vi "UMLEditor reversedEngineering.vi"(1 "AddProjectClasses":bool, 2 "ClassToAnalyse/XMI File To Read":path, 3 "XMI Import":bool, 5 "error in (no error)":errorcluster) -> (16 "cancel":bool, 17 "newCLassDiagram":refnum<class "Graph.lvclass">, 19 "error out":errorcluster)   [LabVIEW 2020]
doc: "Gets current diagram values"
uses:
  <resource>/Framework/Providers/Open_GDS/UML/UMLEditor/UMLEditor RevEngLocalvarType.ctl
  <resource>/Framework/Providers/Open_GDS/UML/Graph_class/Graph.lvclass
  <resource>/Framework/Providers/Open_GDS/UML/Graphics_class/Graphics.lvclass
  <resource>/Framework/Providers/Open_GDS/UML/Grid_class/Grid.lvclass
  <resource>/Framework/Providers/Open_GDS/UML/ClassNode_class/ClassNode.lvclass
  C:/Program Files (x86)/National Instruments/LabVIEW 2020/resource/Framework/Providers/Open_GDS/UML/RectangularNode_class/RectangularNode.lvclass
  C:/Program Files (x86)/National Instruments/LabVIEW 2020/resource/Framework/Providers/Open_GDS/UML/AbstractNode_class/AbstractNode.lvclass
  <resource>/Framework/Providers/Open_GDS/UML/AbstractEdge_class/AbstractEdge.lvclass
  <resource>/Framework/Providers/Open_GDS/UML/AbstractNode_class/AbstractNode.lvclass
  <resource>/Framework/Providers/Open_GDS/UML/ReversedEngineering/ReversedEngineering ClassInfoType.ctl
  <resource>/Framework/Providers/Open_GDS/UML/UMLEditor/UMLEditor_VisibilityType.ctl
  <resource>/Framework/Providers/Open_GDS/UML/ReversedEngineering/ReversedEngineering AttributeInfoType.ctl
  <resource>/Framework/Providers/Open_GDS/ClassProviders/Common/CommonVIs/CommonVIs_AttributeDataType.ctl
  <resource>/Framework/Providers/Open_GDS/UML/ReversedEngineering/ReversedEngineering_ClassDependencyDetailsType.ctl
  <resource>/Framework/Providers/Open_GDS/ClassProviders/Common/ScriptingFunctions/SubVIs/Scripting_ViDependencyType.ctl
  <resource>/Framework/Providers/Open_GDS/UML/General/Rectangle/Rectangle Rectangle2D.ctl
  <resource>/Framework/Providers/Open_GDS/UML/ReversedEngineering/ReversedEngineering TypeDefType.ctl
  <resource>/Framework/Providers/Open_GDS/UML/ReversedEngineering/ReversedEngineering RecursiveSearchElements.ctl
  <resource>/Framework/Providers/Open_GDS/UML/UMLEditor/UMLEditor_SyncOptions.ctl
  <resource>/Framework/Providers/Open_GDS/UML/UMLEditor/UMLEditor GOOPWizardClassSpecification.ctl
  <resource>/Framework/Providers/Open_GDS/UML/Graphics_class/FontType.ctl
  <resource>/Framework/Providers/Open_GDS/UML/UMLEditor/UMLEditor BusyDialogAction.ctl
  <resource>/Framework/Providers/Open_GDS/UML/ContextHelp/ContextHelp_HelpTexts.ctl
  <resource>/Framework/Providers/Open_GDS/UML/UMLEditor/UMLEditor_StoredPathes.ctl
  <resource>/Framework/Providers/Open_GDS/ClassProviders/Common/File/File_StoredPathesActions.ctl
  <resource>/Framework/Providers/Open_GDS/UML/ClassNode_class/ExternalSetTypes.ctl
  <resource>/Framework/Providers/Open_GDS/UML/ClassRelationshipEdge_class/ExternaSetParamType.ctl
  <resource>/Framework/Providers/Open_GDS/UML/ArrowHead_class/ArrowHeadType.ctl
  <resource>/Framework/Providers/Open_GDS/UML/BentStyle_class/BentStyleType.ctl
  <resource>/Framework/Providers/Open_GDS/UML/Graphics_class/LvFontType.ctl
  <resource>/Framework/Providers/Open_GDS/UML/SegmentedLineEdge_class/SegmentedLineEdge.lvclass
  <resource>/Framework/Providers/Open_GDS/UML/InterfaceNode_class/InterfaceNode.lvclass
  C:/Program Files (x86)/National Instruments/LabVIEW 2020/resource/Framework/Providers/Open_GDS/UML/ClassNode_class/ClassNode.lvclass
  <resource>/Framework/Providers/Open_GDS/UML/ClassRelationshipEdge_class/ClassRelationshipEdge.lvclass
  C:/Program Files (x86)/National Instruments/LabVIEW 2020/resource/Framework/Providers/Open_GDS/UML/AbstractEdge_class/AbstractEdge.lvclass
  <resource>/Framework/Providers/Open_GDS/UML/ClassDiagramGraph_class/ClassDiagramGraph.lvclass
  C:/Program Files (x86)/National Instruments/LabVIEW 2020/resource/Framework/Providers/Open_GDS/UML/Graph_class/Graph.lvclass
  <resource>/Framework/Providers/Open_GDS/UML/ArrowHead_class/ArrowHead.lvclass
  <resource>/Framework/Providers/Open_GDS/UML/BentStyle_class/BentStyle.lvclass
  <resource>/Framework/Providers/Open_GDS/UML/RectangularNode_class/RectangularNode.lvclass
  <resource>/Framework/Providers/Open_GDS/UML/UmlEditor_class/UmlEditor.lvclass
panel:
  in  "SyncOption":T1
  in  "AddDirsRec":bool
  in  "ReverseCurrectProject":bool
  out "SearchElements":T2[](array[typedef])
  in  "Remove":bool
  in  "ClearList":bool
  in  "AddDirs":bool
  in  "AddClasses":bool
  in  "AddTopVIs":bool
  in  "Pathes":i32[](listbox) caption="Top VIs, Classes(llbs/dirs) and Directories that should be analysed"
  out "ApplicationNodes":i32[](array[numeric])
  in  "CreateApplication":bool caption="Create Main Application Node"
  in  "Help":bool
  in  "OnlyInheritance":bool caption="Only Create Inheritance classes"
  in  "CreateTypes":bool caption="Create TypeDefs"
  in  "HideSubAss":bool=TRUE caption="Hide SubClass assosiates to classes that BaseClass already associates to"
  in  "screenRef":refnum<vi>
  out "files":path[](array[path])
  in  "cancel":bool
  in  "ok":bool
  in  "local":T3 {"block"."bounds"."height" format="%.2f"; "block"."bounds"."width" format="%.2f"; "block"."bounds"."y" format="%.2f"; "block"."bounds"."x" format="%.2f"; "bounds"."height" format="%.2f"; "bounds"."width" format="%.2f"; "bounds"."y" format="%.2f"; "bounds"."x" format="%.2f"}
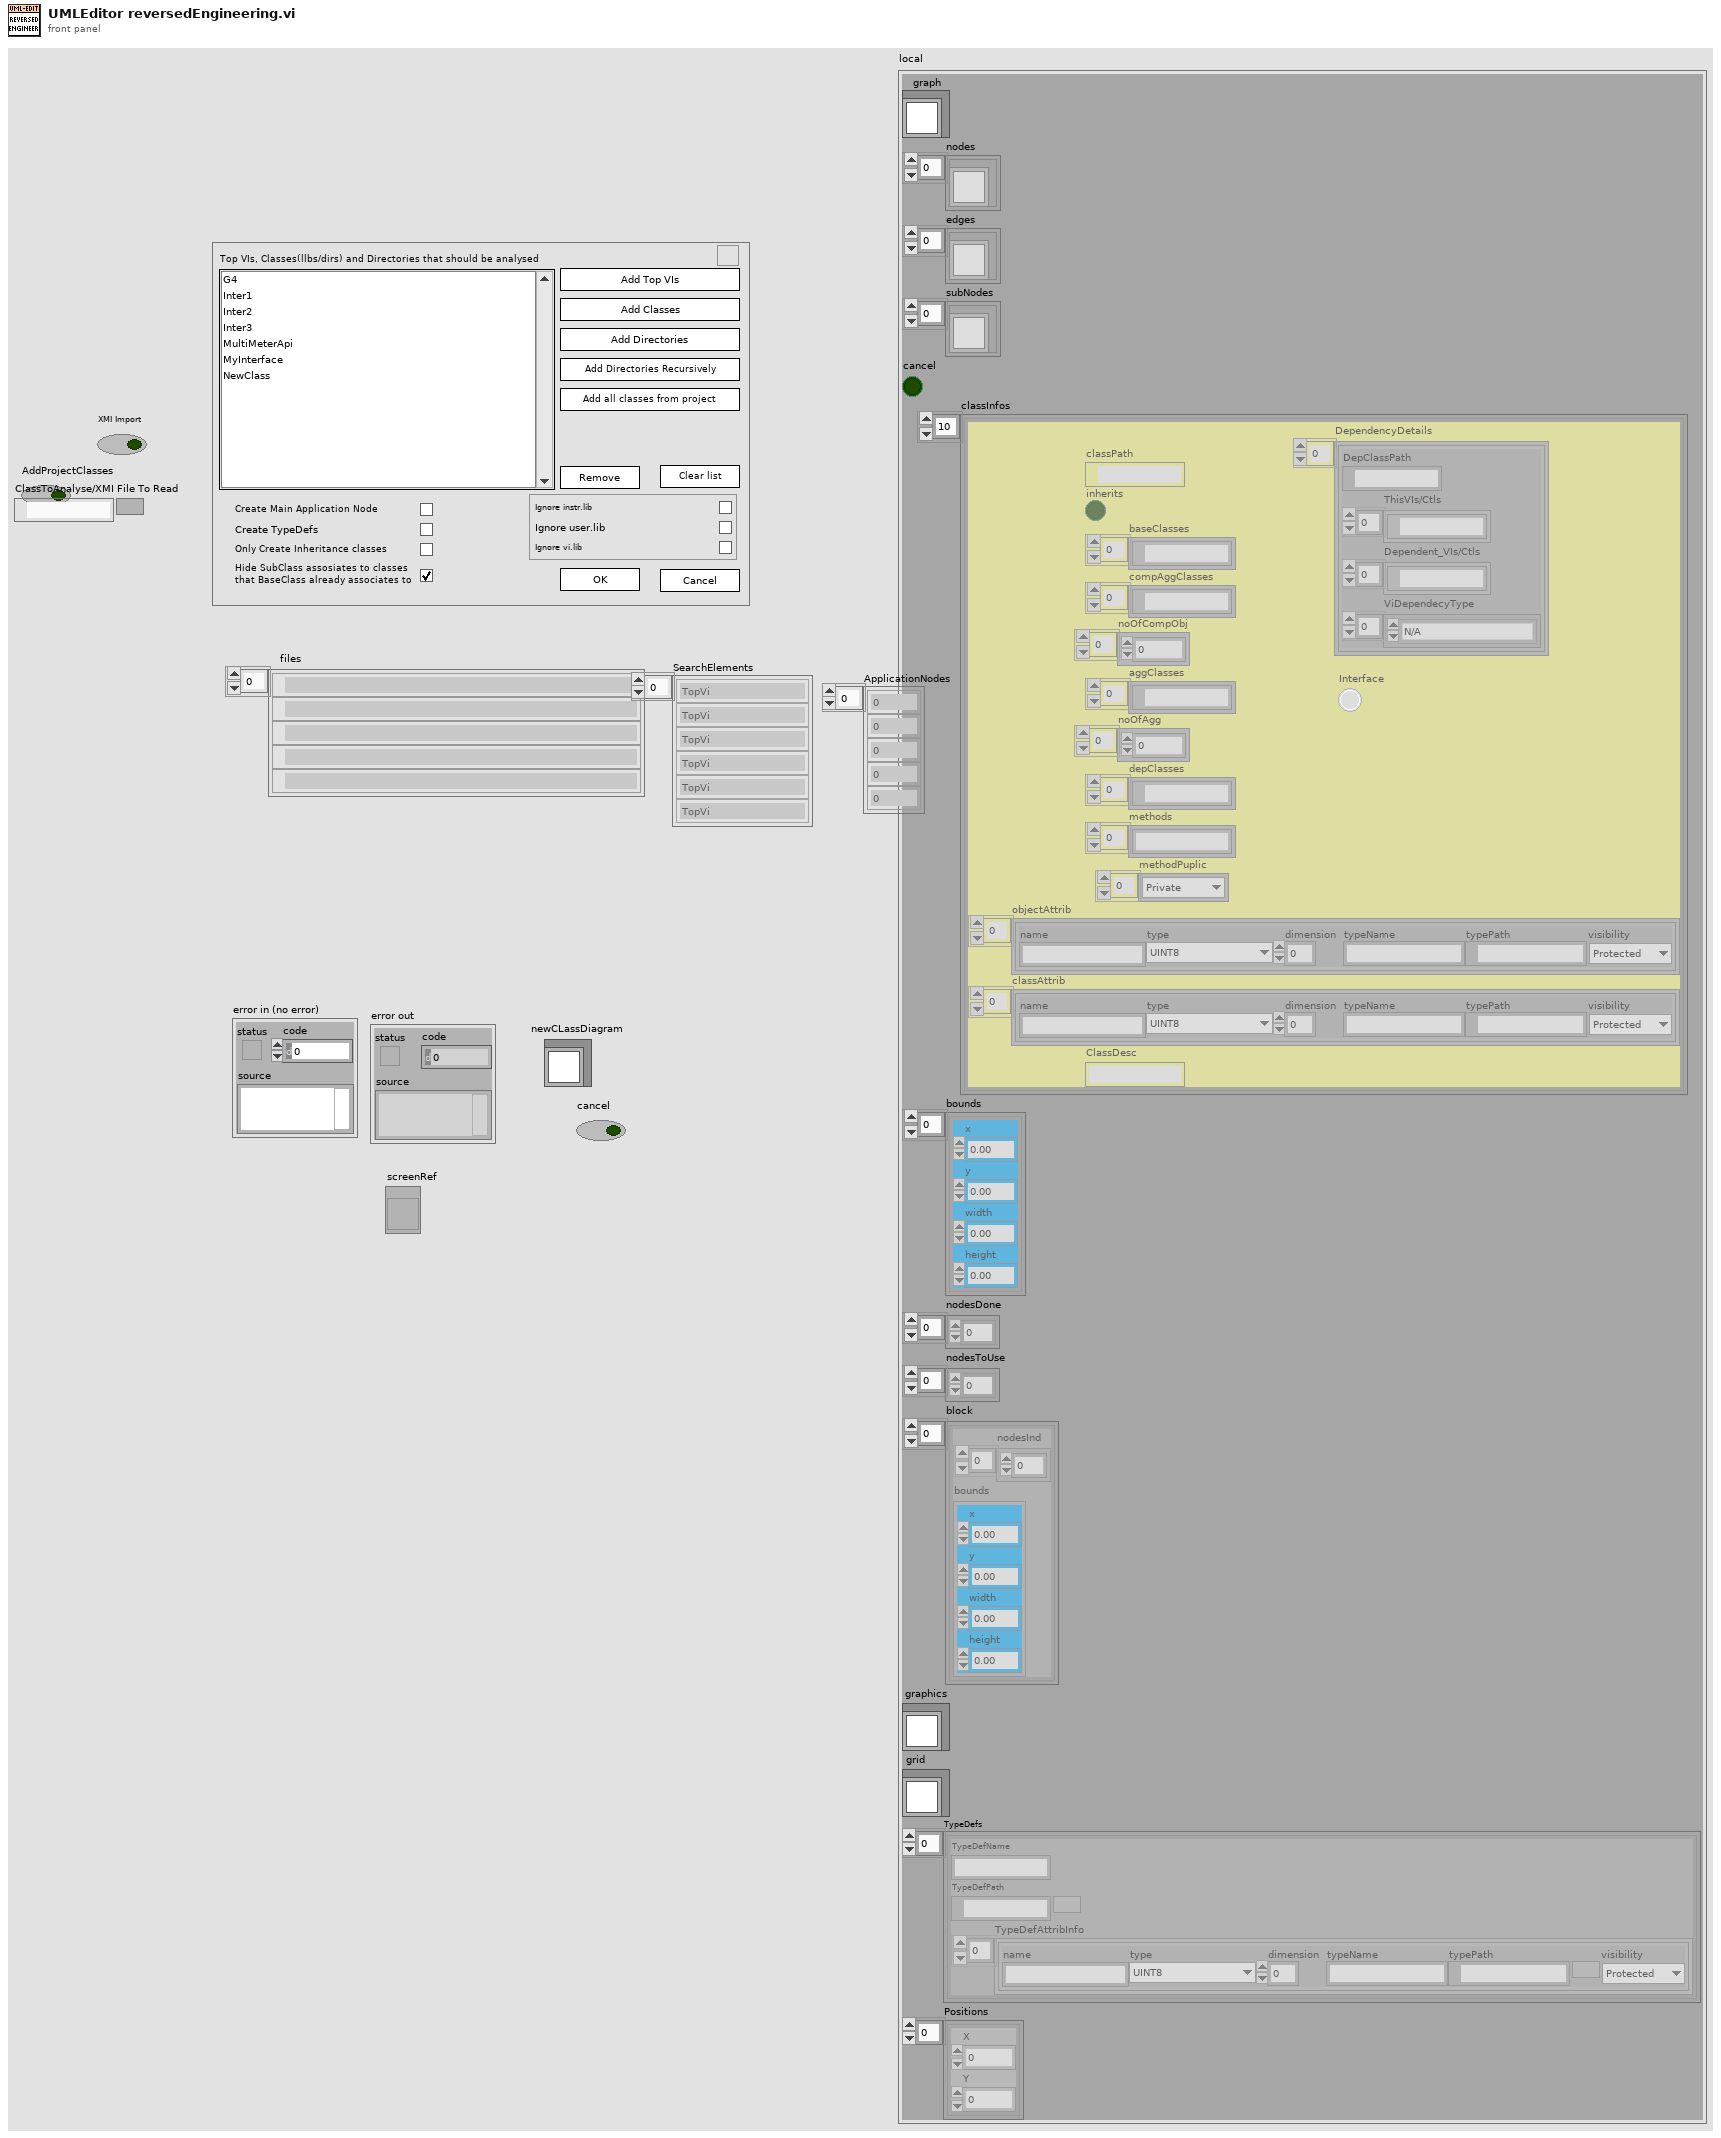
[diagram p1: front panel]
types:
  T1 = typedef "UMLEditor_SyncOptions.ctl" = cluster{"IgnoreInstrLib":bool, "IgnoreUserLib":bool, "IgnoreViLib":bool}
  T2 = typedef "ReversedEngineering RecursiveSearchElements.ctl" = enum16{"TopVi", "Class", "Dir", "Dir(rec.)"}
  T3 = typedef "UMLEditor RevEngLocalvarType.ctl" = cluster{"graph":refnum<class "Graph.lvclass">, "nodes":refnum<class "ClassNode.lvclass">[], "edges":refnum<class "AbstractEdge.lvclass">[], "subNodes":refnum<class "AbstractNode.lvclass">[], "cancel":bool, "classInfos":T4[], "bounds":T10[], "nodesDone":i32[], "nodesToUse":i32[], "block":cluster{"nodesInd":i32[], "bounds":T10}[], "graphics":refnum<class "Graphics.lvclass">, "grid":refnum<class "Grid.lvclass">, "TypeDefs":T11[], "Positions":cluster{"X":i32, "Y":i32}[]}
  T4 = typedef "ReversedEngineering ClassInfoType.ctl" = cluster{"classPath":path, "inherits":bool, "baseClasses":path[], "compAggClasses":path[], "noOfCompObj":i32[], "aggClasses":path[], "noOfAgg":i32[], "depClasses":path[], "methods":string[], "methodPuplic":T5[], "objectAttrib":T6[], "classAttrib":T6[], "ClassDesc":string, "DependencyDetails":T8[], "Interface":bool}
  T5 = typedef "UMLEditor_VisibilityType.ctl" = enum16{"Public", "Private", "Protected"}
  T6 = typedef "ReversedEngineering AttributeInfoType.ctl" = cluster{"name":string, "type":T7, "dimension":i32, "typeName":string, "typePath":path, "visibility":T5}
  T7 = typedef "CommonVIs_AttributeDataType.ctl" = enum16{"UINT8", "INT8", "UINT16", "INT16", "UINT32", "INT32", "UINT64", "INT64", "SGL", "DBL", "EXT", "CSG", "CDB", "CXT", "TimeStamp", "STRING", "PATH", "BOOL", "ENUM", "RefNum", "VIRefNum", "LabVIEW Class", "Cluster", "Variant", "TypeDef", "Waveform", "LabVIEW Object", "Other", "void"}
  T8 = typedef "ReversedEngineering_ClassDependencyDetailsType.ctl" = cluster{"DepClassPath":path, "ThisVIs/Ctls":path[], "Dependent_VIs/Ctls":path[], "ViDependecyType":T9[]}
  T9 = typedef "Scripting_ViDependencyType.ctl" = enum16{"N/A", "Launches"}
  T10 = typedef "Rectangle Rectangle2D.ctl" = cluster{"x":dbl, "y":dbl, "width":dbl, "height":dbl}
  T11 = typedef "ReversedEngineering TypeDefType.ctl" = cluster{"TypeDefName":string, "TypeDefPath":path, "TypeDefAttribInfo":T6[]}
  T12 = typedef "UMLEditor BusyDialogAction.ctl" = enum16{"Initialize", "Open(VIs)", "Open(i)", "Send_I-Value", "SendStatusMessage", "GetBusyDialogStatus", "Close", "Quit"}
  T13 = typedef "Graphics.lvclass/FontType.ctl" = cluster{"Font Name:":string, "Size":i16, "Strikeout?":bool, "Italic?":bool, "Underline?":bool, "Outline?":bool, "Shadow?":bool, "Bold?":bool}
  T14 = typedef "UMLEditor GOOPWizardClassSpecification.ctl" = cluster{"ClassName":string, "Class folder":path, "ClassType":i32, "LLB":bool, "Base class":path, "SeparatorChar":string, "Class description":string, "ClassIconInfo":cluster{"Icon class name":string, "Frame color":u32, "Header color":u32, "Public color":u32, "Private color":u32, "Foreground color":u32, "Protected color":u32}, "Methods":cluster{"MethodName":string, "Private":bool, "Virtual":bool, "Protected":bool, "Method Type":i32, "Description":string, "Icon Method Name":string}[], "VirtualMethods":bool, "BaseClass":bool, "ClassStereotype":string, "ExistsAsFile":bool, "ExistsInProject":bool, "ClassTemplateOption":string, "LVClassRef":refnum<vi>, "Node":refnum<class "ClassNode.lvclass">}
  T15 = typedef "ContextHelp_HelpTexts.ctl" = enum16{"None(Hide)", "Default", "Help", "Welcome", "GettingStarted", "ClassDiagram_Help", "SequenceDiagram_Help", "UseCaseDiagram_Help", "BSelect", "BClass", "BInterface", "BPackage", "BNote", "BDependency", "BInheritance", "BInterfaceImplementation", "BAssociation", "BAggregation", "BCompAggregation", "BNoteConnector", "BObject", "BActionBar", "BCall", "BSystem", "BActor", "BUseCase", "BGeneralization", "BIncludes", "BExtends", "BUseCaseDiagramAssociation", "ClassRelationshipEdge editDialog_Bent Style", "ClassRelationshipEdge editDialog_RelationType", "ClassRelationshipEdge editDialog_Reverse association", "ClassRelationshipEdge editDialog_Start label", "ClassRelationshipEdge editDialog_Middle label", "ClassRelationshipEdge editDialog_End label", "UMLEditor reversedEngineering_Pathes", "ReversedEngineering StateReverseDialog_Help", "ReversedEngineering StateQueuedSettings_Help", "UMLEditor reversedEngineering_AddTopVIs", "UMLEditor reversedEngineering_AddClasses", "UMLEditor reversedEngineering_AddDirs", "UMLEditor reversedEngineering_Recursively", "UMLEditor reversedEngineering_Remove", "UMLEditor reversedEngineering_ClearList", "UMLEditor reversedEngineering_HideSubAss", "UMLEditor reversedEngineering_CreateTypes", "UMLEditor reversedEngineering_OnlyInheritance", "UMLEditor reversedEngineering_CreateApplication", "UMLEditor reversedEngineering_OK", "UMLEditor reversedEngineering_Cancel", "UMLEditor reversedEngineering_Help", "UMLEditor createWizardScriptFile_ScriptfilePath", "UMLEditor createWizardScriptFile_ClassPath", "UMLEditor createWizardScriptFile_Use", "UMLEditor createWizardScriptFile_PrivateDirName", "UMLEditor createWizardScriptFile_DirAppend", "UMLEditor createWizardScriptFile_Separator Character", "UMLEditor createWizardScriptFile_OK", "UMLEditor createWizardScriptFile_Cancel", "UMLEditor createWizardScriptFile_Help", "ClassNode editDialog_Class Name", "InterfaceNode editDialog_Class Name", "ClassNode editDialog_Attribute", "ClassNode editDialog_Methods", "InterfaceNode editDialog_Methods", "ClassNode editDialog_connection", "InterfaceNode editDialog_connection", "ClassNode editDialog_StereoType", "ClassNode editDialog_ShowAttrib", "ClassNode editDialog_ShowMethods", "ClassNode editDialog_ClassPath", "ClassNode editDialog_AddAttribute", "ClassNode editDialog_AddMethod", "InterfaceNode editDialog_AddMethod", "ClassNode AttributeGuide_AttributeName", "ClassNode AttributeGuide_Array?", "ClassNode AttributeGuide_Data Type", "ClassNode AttributeGuide_RefName", "ClassNode AttributeGuide_Preview", "ClassNode AttributeGuide_OK", "ClassNode AttributeGuide_Cancel", "ClassNode MethodGuide_Visibility", "ClassNode MethodGuide_Method Name", "ClassNode MethodGuide_Preview", "ClassNode MethodGuide_OK", "ClassNode MethodGuide_Cancel", "CallNode EditCallProperties_AllButtons", "ObjectNode EditObjectlProperties_AllButtons", "ActorNode EditActorProperties_AllButtons", "UseCaseRelationshipNode EditUseCaselProperties_AllButtons", "UseCaseNode EditUseCaselProperties_AllButtons", "SystemNode EditSystemProperties_AllButtons", "ReversedEngineering UpdateAttributes_AllButtons", "StateNode editDialog_AllButtons", "StateTransition editDialog_AllButtons", "ArrangeNodes Main_Picture", "ArrangeNodes Main_Zoom", "ArrangeNodes Main_Auto Zoom", "ArrangeNodes Main_shorten", "ArrangeNodes Main_Min Length", "ArrangeNodes Main_Max Length", "ArrangeNodes Main_increase", "ArrangeNodes Main_decrease", "ArrangeNodes Main_Shake", "ArrangeNodes Main", "BState", "BInitialState", "BFinalState", "BStateTransition", "StateDiagram_Help", "StateDiagram_PropertiesAllButtons", "ReversedEngineering StateReverseDialog_ClearStates", "ReversedEngineering StateReverseDialog_UseQueuedStateMachines", "ReversedEngineering StateReverseDialog_QueuedSettings", "ReversedEngineering StateReverseDialog_SearchForVIs", "ReversedEngineering StateReverseDialog_SearchCriteria", "OptionsDialog_ClassBasePath", "OptionsDialog_VIPath", "OptionsDialog_ApplicationPath", "OptionsDialog_WizDir", "OptionsDialog_IniFilePath", "OptionsDialog_DefineColors", "OptionsDialog_Help", "OptionsDialog_CreateTypes", "ClassRelationshipEdge editDialog_SplitWire"}
  T16 = typedef "File_StoredPathesActions.ctl" = enum16{"Get Path", "Set Path", "Delete Path", "Clear All Paths"}
  T17 = enum32{"existing file", "new file", "new or existing file", "existing dir", "new dir", "new or existing dir", "existing file (use LLBs)", "new file (use LLBs)", "new or existing file (use LLBs)", "new or existing file or directory (use LLBs)"}
  T18 = enum8{"Enabled", "Disabled", "Disabled and Grayed Out"}
  T19 = typedef "ClassNode.lvclass/ExternalSetTypes.ctl" = enum16{"Name", "Attributes", "Methods", "Position", "ShowMethods", "ShowAttributes", "ClassPath"}
  T20 = typedef "BentStyle.lvclass/BentStyleType.ctl" = enum16{"STRAIGHT", "HV", "VH", "HVH", "VHV", "ARC"}
  T21 = typedef "ClassRelationshipEdge.lvclass/ExternaSetParamType.ctl" = enum16{"StartLabel", "MidLabel", "EndLabel", "StartNode", "EndNode", "BendType", "StartArrow", "EndArrow"}
  T22 = typedef "ArrowHead.lvclass/ArrowHeadType.ctl" = enum16{"NONE", "TRIANGLE", "BLACK_TRIANGLE", "V", "HALF_V", "DIAMOND", "BLACK_DIAMOND"}
  T23 = typedef "Graphics.lvclass/LvFontType.ctl" = enum16{"User-specified Font", "Application Font", "System Font", "Dialog Font"}
  T24 = typedef "ContextHelp_ShowType.ctl" = cluster{"Header":string, "Picture":picture, "Text":string}
  T25 = typedef "UMLEditor_StoredPathes.ctl" = enum16{"LastSearchPath", "QueuedArrayStateVI", "ClassBasePath", "ViTemplatePath", "ApplicationTemplatePath", "IniFilePath", "WizDir", "RevPlugInPath"}
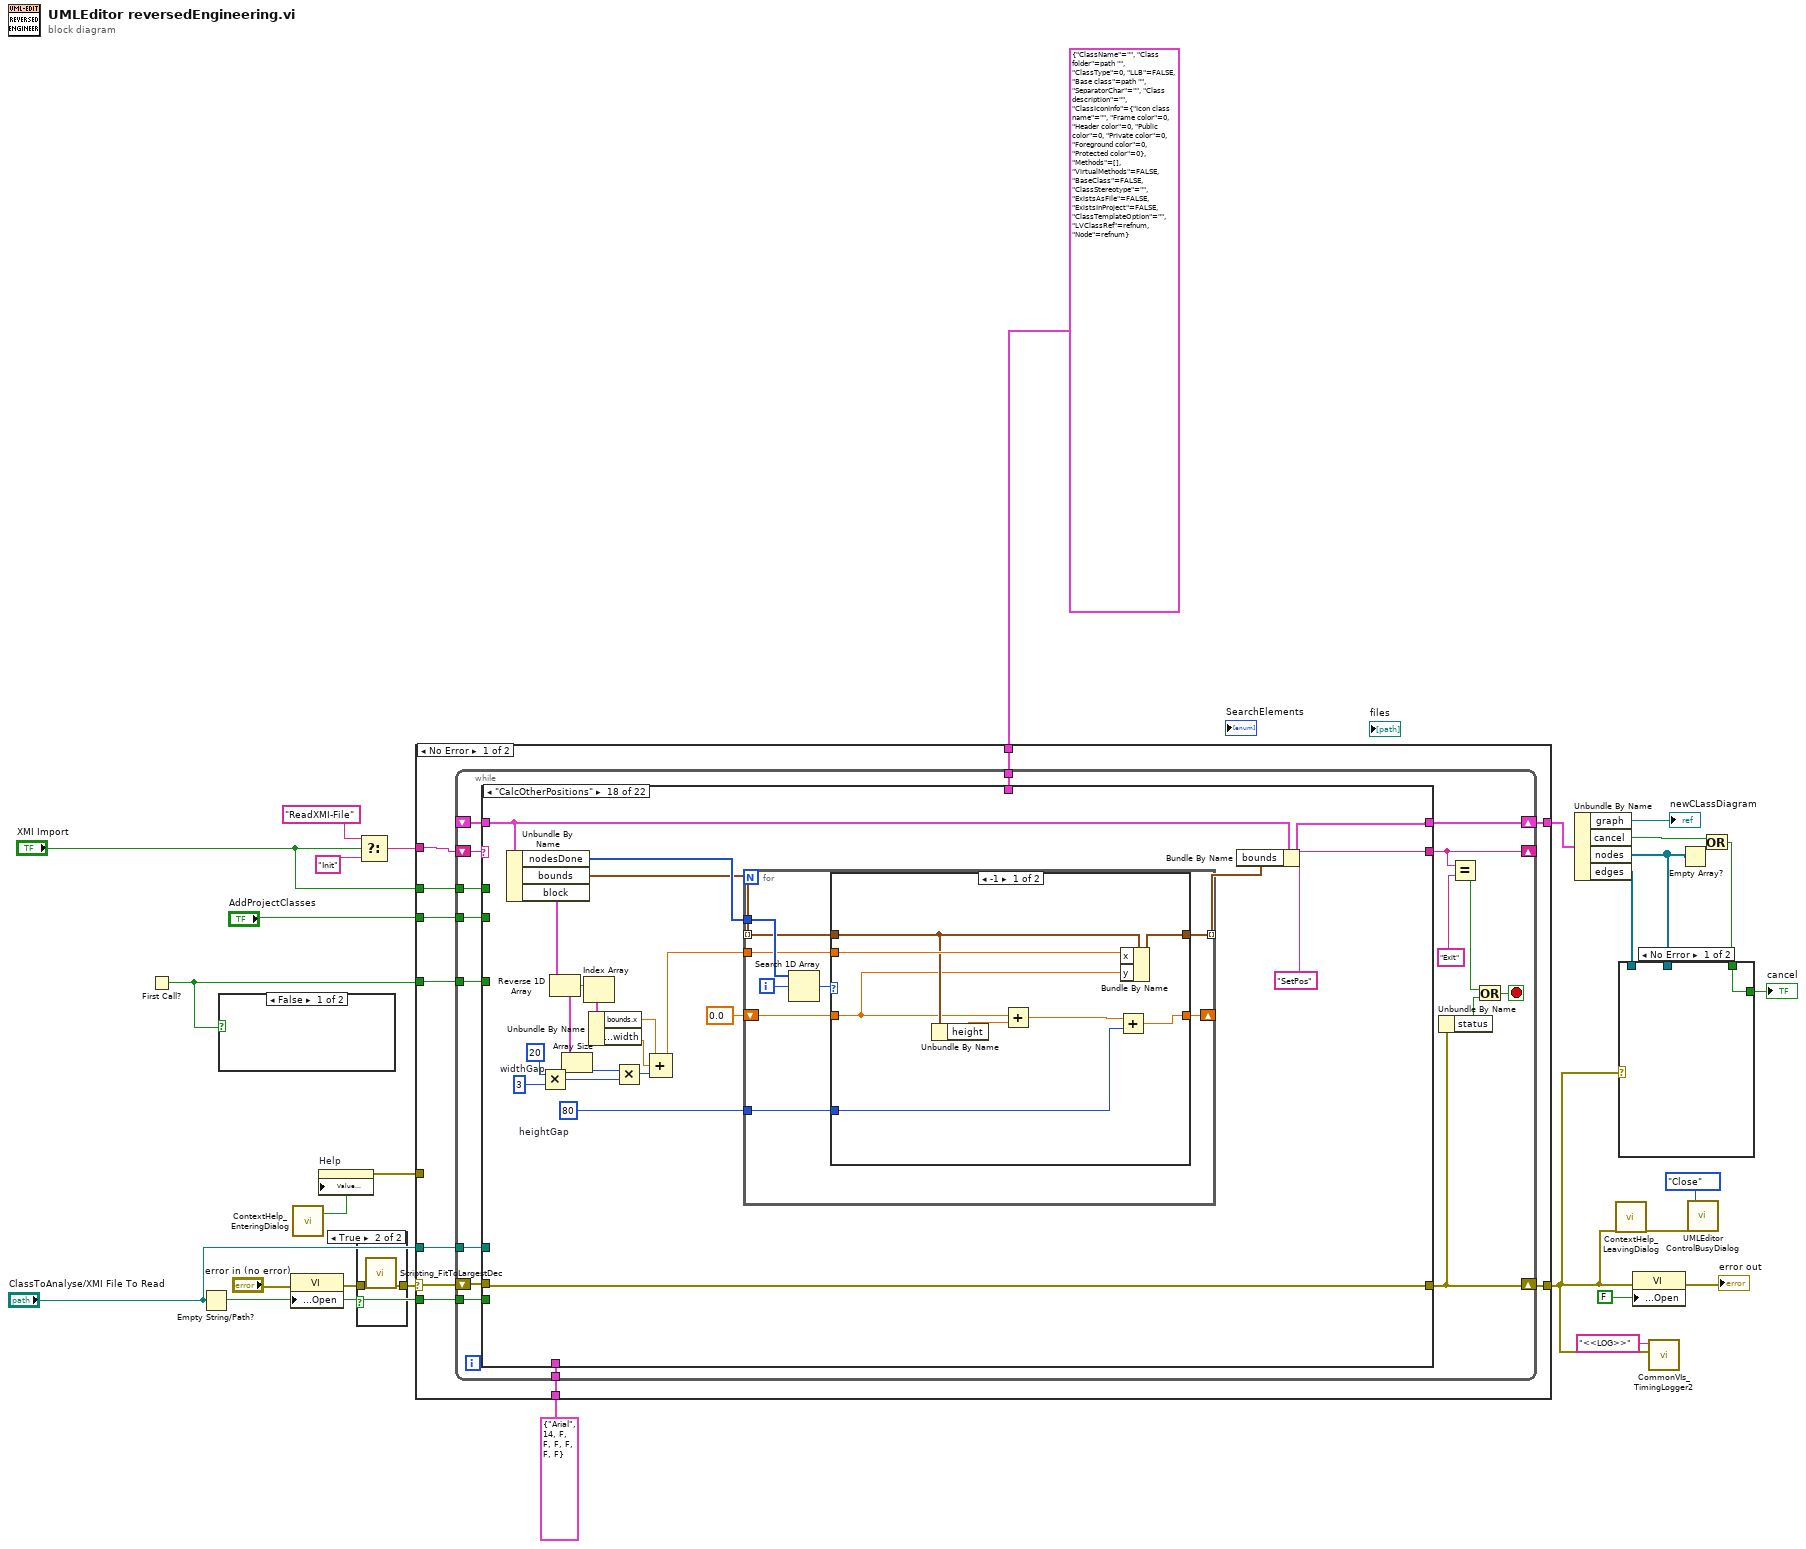
[diagram p0: block diagram]
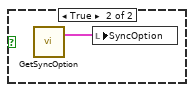
[diagram p2: hidden frame]
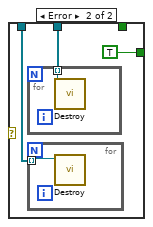
[diagram p4: hidden frame]
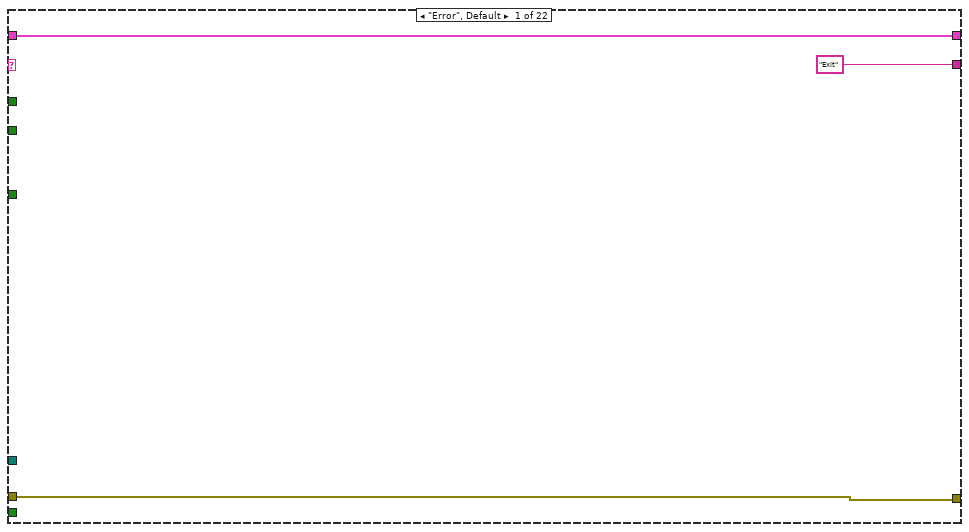
[diagram p5: hidden frame]
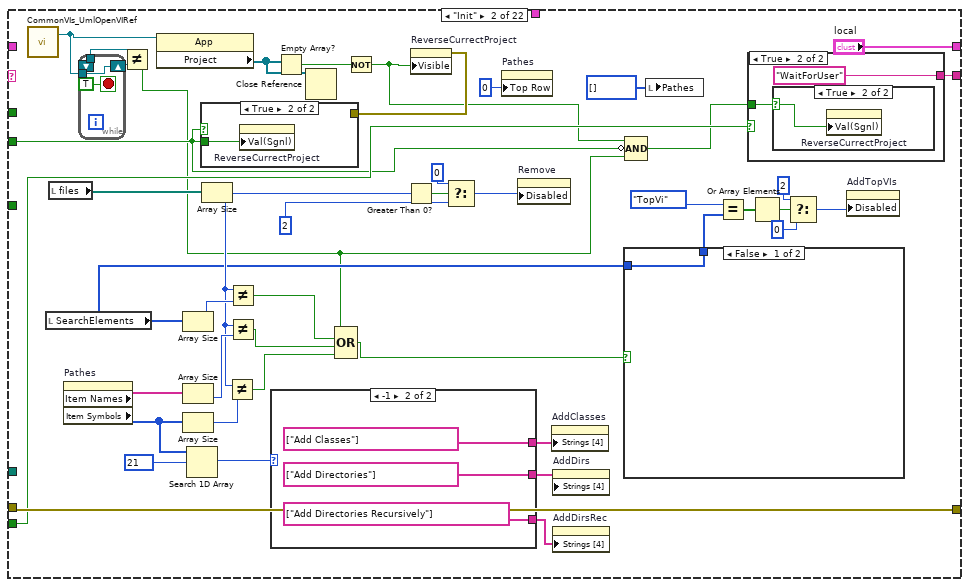
[diagram p6: hidden frame]
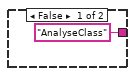
[diagram p7: hidden frame]
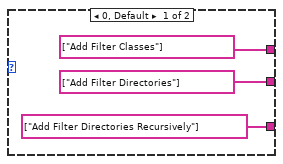
[diagram p10: hidden frame]
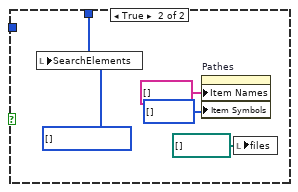
[diagram p11: hidden frame]
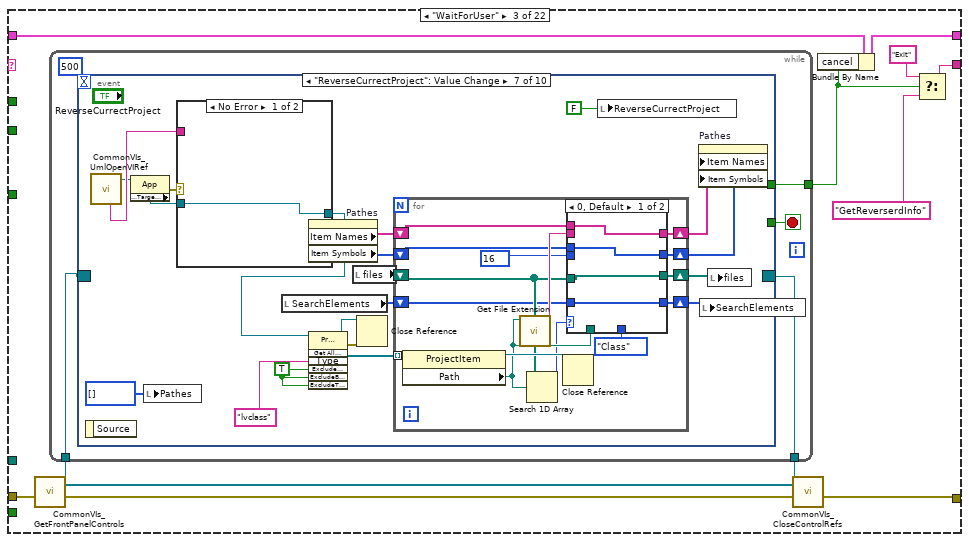
[diagram p12: hidden frame]
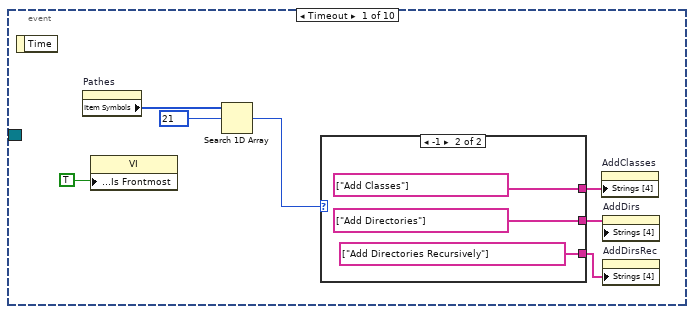
[diagram p13: hidden frame]
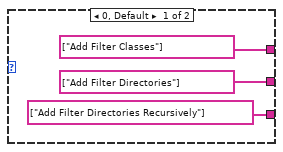
[diagram p14: hidden frame]
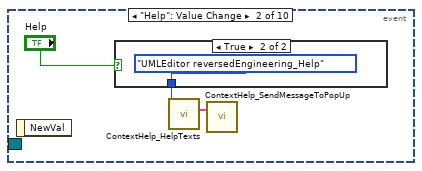
[diagram p15: hidden frame]
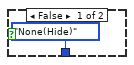
[diagram p16: hidden frame]
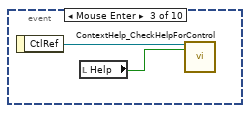
[diagram p17: hidden frame]
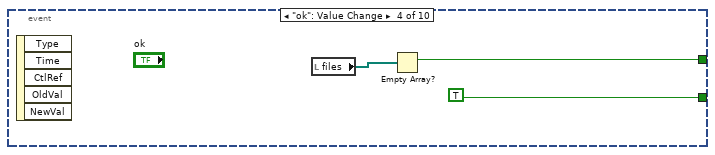
[diagram p18: hidden frame]
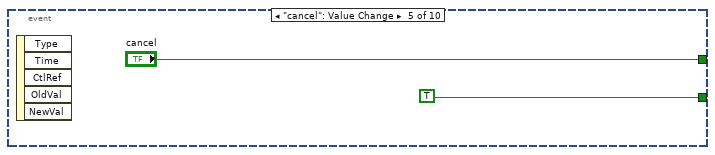
[diagram p19: hidden frame]
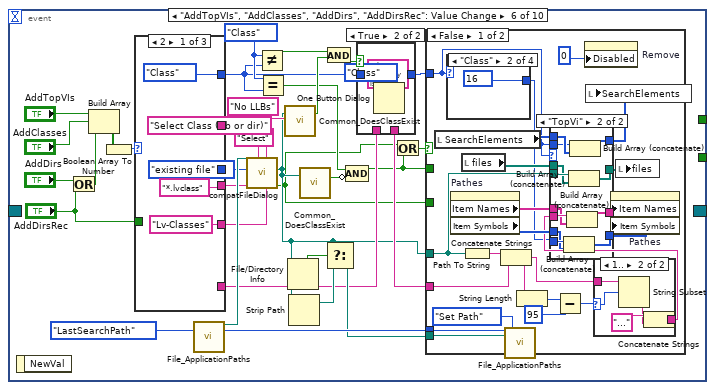
[diagram p20: hidden frame]
diagram:
  n1 = First Call?() -> (First Call?: T/F=w7:bool)
  n2 = Empty String/Path?(string/path="ClassToAnalyse/XMI File To Read") -> (empty?=w8:bool)
  n3 = case shown="False" w7 {
    frame False {
    }
    frame True {
      n4 = call <resource>:"GetSyncOption.vi"() -> ("SyncOption"=w30:T1)  [unwired: 17 in, 2 out]
      n5 = local write "SyncOption"(w30) -> ()
    }
  }
  n6 = property class="VI"(error in="error in (no error)", "Front Panel.Open"=w8) -> (error out=w10:errorcluster)  [unwired: 1 in, 1 out]
  n7 = call <resource>:"ContextHelp_EnteringDialog.vi"() -> ("HelpStatus"=w23:bool)  [unwired: 1 in, 18 out]
  n8 = property on="Help" class="Bool (strict)"("Value (Signaling)"=w23) -> (error out=w22:errorcluster)  [unwired: 2 in, 1 out]
  n9 = case shown="True" w8 {
    tunnel: w10 -> [w31 w33]
    tunnel: [w31 w32] -> w9
    frame False {
    }
    frame True {
      n10 = call <resource>:"Scripting_FitToLargestDec.vi"("error in (no error)"=w33) -> ("error out"=w32:errorcluster)  [unwired: 5 in, 1 out]
    }
  }
  n11 = Select(t="ReadXMI-File", s="XMI Import", f="Init") -> (s? t:f=w5:string)
  n12 = case shown="No Error" w9 {
    selector: w9 -> [w43 w1191]
    tunnel: [w44 w1191] -> w2
    tunnel: T14 {"ClassName"="", "Class folder"=path "", "ClassType"=0, "LLB"=FALSE, "Base class"=path "", "SeparatorChar"="", "Class description"="", "ClassIconInfo"={"Icon class name"="", "Frame color"=0, "Header color"=0, "Public color"=0, "Private color"=0, "Foreground color"=0, "Protected color"=0}, "Methods"=[], "VirtualMethods"=FALSE, "BaseClass"=FALSE, "ClassStereotype"="", "ExistsAsFile"=FALSE, "ExistsInProject"=FALSE, "ClassTemplateOption"="", "LVClassRef"=refnum, "Node"=refnum} ("Class Info") -> [w42 _]
    tunnel: [w41 _] -> w28
    tunnel: w7 -> [w40 _]
    tunnel: w22 -> [_ _]
    tunnel: T13 {"Font Name:"="Arial", "Size"=14, "Strikeout?"=FALSE, "Italic?"=FALSE, "Underline?"=FALSE, "Outline?"=FALSE, "Shadow?"=FALSE, "Bold?"=FALSE} ("font") -> [w39 _]
    tunnel: "AddProjectClasses" -> [w38 _]
    tunnel: w8 -> [w37 _]
    tunnel: "ClassToAnalyse/XMI File To Read" -> [w36 _]
    tunnel: w5 -> [w35 _]
    tunnel: "XMI Import" -> [w34 _]
    frame No Error {
      n13 = while {
        shift-right: [w57] -> w44
        shift-left: w43 -> [w61]
        shift-right: [w55] -> _
        shift-left: w35 -> [w60]
        shift-right: [w59] -> w41
        shift-left: _ -> [w58]
        tunnel: w42 -> [w51]
        tunnel: w40 -> [w50]
        tunnel: w39 -> [w49]
        tunnel: w38 -> [w48]
        tunnel: w37 -> [w47]
        tunnel: w36 -> [w46]
        tunnel: w34 -> [w45]
        stop <- w52 stop-if-true
        n14 = case shown="\"CalcOtherPositions\"" w60 {
          tunnel: w61 -> [w62 w107 w137 w403 w433 w460 w465 w521 w568 w649 w686 w744 w766 w834 w901 w950 w1020 w1032 w1073 w1101 w1170 w1183]
          tunnel: [w62 w107 w137 w403 w426 w456 w465 w521 w566 w649 w678 w737 w753 w822 w880 w950 w992 w1032 w1066 w1095 w1156 w1182] -> w57
          tunnel: [w63 "local" w132 w404 w449 w455 w471 w509 w577 w652 w684 w740 w765 w833 w905 w951 w1025 w1046 w1075 w1111 w1162 w1184] -> w59
          tunnel: ["Exit" w108 w135 "GetReverserdInfo" ("f") w421 "CreateNodes" ("y") w461 "CreateNodes" ("y") "RemoveDubbleTypeDefs" "CreateTypeDefsNodes" "CreateEdges" "CreateTypeDefEdgesFromClasses" "CreateTypeDefEdgesFromTypeDefs" "GetBounds" "CheckInheritance" ("y") w942 "CheckInheritance" ("y") "SetPos" ("y") "TranslateAplicationNodes?" ("y") "CreateDiagram" ("y") w1166 "Exit" ("y")] -> w55
          tunnel: w58 -> [w63 _ w133 w404 w448 w459 w469 w511 w578 w653 w683 w741 w763 w831 w904 w947 w1019 w1037 w1075 w1111 w1168 w1184]
          tunnel: w51 -> [_ _ _ _ _ _ _ _ _ _ _ _ _ _ _ _ _ _ _ _ _ _]
          tunnel: w50 -> [_ _ _ _ _ _ _ _ _ _ _ _ _ _ _ _ _ _ _ _ _ _]
          tunnel: w49 -> [_ _ _ _ _ _ _ _ _ _ _ _ _ _ w893 _ _ _ _ _ _ _]
          tunnel: w48 -> [_ w69 _ _ _ _ _ _ _ _ _ _ _ _ _ _ _ _ _ _ _ _]
          tunnel: w47 -> [_ w77 _ _ w420 _ _ _ _ _ _ _ _ _ _ _ _ _ _ _ _ _]
          tunnel: w46 -> [_ _ _ w398 _ w454 _ _ _ _ _ _ _ _ _ _ _ _ _ _ _ _]
          tunnel: w45 -> [_ _ _ _ _ _ _ _ _ _ _ _ _ _ _ _ _ _ _ _ w1159 _]
          frame "Error", Default {
          }
          frame "Init" {
            n15 = call <resource>:"CommonVIs_UmlOpenVIRef.vi"() -> ("AppRefOut"=w66:refnum<vi>)  [unwired: 4 in, 7 out]
            n16 = local read "SearchElements"() -> (w79:T2[])
            n17 = local read "files"() -> (w105:path[])
            n18 = property on="Pathes" class="LstBox (strict)"() -> ("Item Names"=w103:string[], "Item Symbols"=w91:i32[])  [unwired: 2 in, 2 out]
            n19 = while {
              shift-right: [w110] -> w74
              shift-left: _ -> [w109]
              tunnel: w66 -> [w110]
              tunnel: [w109] -> w73
              stop <- TRUE stop-if-true
            }
            n20 = Not Equal?(x=w73, y=w74) -> (x != y?=w68:bool)
            n21 = property class="App"(reference=w66) -> ("Project"=w72:refnum<vi>[])  [unwired: 1 in, 2 out]
            n22 = Array Size(array=w79) -> (size(s)=w104:i32)
            n23 = Array Size(array=w103) -> (size(s)=w102:i32)
            n24 = Array Size(array=w91) -> (size(s)=w101:i32)
            n25 = Search 1D Array(1D array=w91, element=21) -> (index of element=w89:i32)  [unwired: 1 out]
            n26 = Array Size(array=w105) -> (size(s)=w96:i32)
            n27 = Not Equal?(x=w96, y=w101) -> (x != y?=w98:bool)
            n28 = Not Equal?(x=w96, y=w104) -> (x != y?=w100:bool)
            n29 = Not Equal?(x=w96, y=w102) -> (x != y?=w99:bool)
            n30 = case shown="-1" w89 {
              tunnel: [string[] ["Add Filter Classes"] ("Strings [4]") string[] ["Add Classes"] ("Strings [4]")] -> w88
              tunnel: [string[] ["Add Filter Directories"] ("Strings [4]") string[] ["Add Directories"] ("Strings [4]")] -> w87
              tunnel: [string[] ["Add Filter Directories Recursively"] ("Strings [4]") string[] ["Add Directories Recursively"] ("Strings [4]")] -> w75
              frame 0, Default {
              }
              frame -1 {
              }
            }
            n31 = Empty Array?(array=w72) -> (empty?=w78:bool)
            n32 = Close Reference(reference=w72) -> ()  [unwired: 1 in, 1 out]
            n33 = Compound Arithmetic op=OR(w68, w100, w99, w98) -> (w97:bool)
            n34 = Not(x=w78) -> (.not. x?=w70:bool)
            n35 = Greater Than 0?(x=w96) -> (x > 0?=w95:bool)
            n36 = property on="ReverseCurrectProject" class="Bool (strict)"("Visible"=w70) -> (error out=w71:errorcluster)  [unwired: 2 in, 1 out]
            n37 = case shown="True" w69 {
              tunnel: w69 -> [_ w116]
              tunnel: w71 -> [_ _]
              frame False {
              }
              frame True {
                n38 = property on="ReverseCurrectProject" class="Bool (strict)"("Val(Sgnl)"=w116) -> ()  [unwired: 2 in, 2 out]
              }
            }
            n39 = Select(t=u8 0 ("Disabled"), s=w95, f=u8 2 ("Disabled")) -> (s? t:f=w94:u8)
            n40 = property on="Pathes" class="LstBox (strict)"("Top Row"=0) -> ()  [unwired: 2 in, 2 out]
            n41 = property on="Remove" class="Bool"("Disabled"=w94) -> ()  [unwired: 2 in, 2 out]
            n42 = property on="AddClasses" class="Bool"("Strings [4]"=w88) -> ()  [unwired: 2 in, 2 out]
            n43 = property on="AddDirs" class="Bool"("Strings [4]"=w87) -> ()  [unwired: 2 in, 2 out]
            n44 = property on="AddDirsRec" class="Bool"("Strings [4]"=w75) -> ()  [unwired: 2 in, 2 out]
            n45 = case shown="False" w97 {
              tunnel: [w123 w124] -> w81
              tunnel: w79 -> [w123 _]
              frame False {
              }
              frame True {
                w124 = T2[] [] items=["TopVi", "Class", "Dir", "Dir(rec.)"] ("SearchElements")
                n46 = local write "SearchElements"(w124) -> ()
                n47 = property on="Pathes" class="LstBox (strict)"("Item Names"=string[] [], "Item Symbols"=i32[] []) -> ()  [unwired: 2 in, 2 out]
                n48 = local write "files"(path[] [] ("files")) -> ()
              }
            }
            n49 = Compound Arithmetic op=AND(w70, invert w69, w68) -> (w67:bool)
            n50 = local write "Pathes"(i32[] [] ("Pathes")) -> ()
            n51 = Equal?(x=ReversedEngineering_RecursiveSearchElements."TopVi" ("deleted portion"), y=w81) -> (x = y?=w86:bool[])
            n52 = case shown="True" w77 {
              tunnel: ["AnalyseClass" ("y") "WaitForUser" ("y")] -> w108
              tunnel: w67 -> [_ w113]
              frame False {
              }
              frame True {
                n53 = case shown="True" w113 {
                  selector: w113 -> [_ w115]
                  frame False {
                  }
                  frame True {
                    n54 = property on="ReverseCurrectProject" class="Bool (strict)"("Val(Sgnl)"=w115) -> ()  [unwired: 2 in, 2 out]
                  }
                }
              }
            }
            n55 = Or Array Elements(Boolean array=w86) -> (logical OR=w85:bool)
            n56 = Select(t=u8 2 ("Disabled"), s=w85, f=u8 0) -> (s? t:f=w83:u8)
            n57 = property on="AddTopVIs" class="Bool"("Disabled"=w83) -> ()  [unwired: 2 in, 2 out]
          }
          frame "WaitForUser" {
            n58 = call <resource>:"CommonVIs_GetFrontPanelControls.vi"() -> ("Event Registration Refnum"=w130:refnum<event-registration>, "ControlRefs"=w128:refnum<vi>[])  [unwired: 2 in, 16 out]
            n59 = while {
              tunnel: [w142] -> w131
              tunnel: w130 -> [w139]
              tunnel: [w138] -> w129
              stop <- w141 stop-if-true
              n60 = event shown="[6] \"ReverseCurrectProject\": Value Change" {
                selector: w139 -> [_ _ _ _ _ _ _ _ _ _]
                dyn-events: [_ _ _ _ _ _ _ _ _ _] -> w138
                timeout: 500 -> [_ _ _ _ _ _ _ _ _ _]
                tunnel: [_ _ _ w163 "cancel" _ _ _ _ _] -> w142
                tunnel: [_ _ _ TRUE ("Front Panel Window:Is Frontmost") TRUE ("Front Panel Window:Is Frontmost") _ _ _ _ _] -> w141
                event Timeout {
                  n61 = event-data() -> ()  [unwired: 2 out]
                  n62 = property on="Pathes" class="LstBox (strict)"() -> ("Item Symbols"=w146:i32[])  [unwired: 2 in, 2 out]
                  n63 = property class="VI"("Front Panel Window:Is Frontmost"=TRUE) -> ()  [unwired: 2 in, 2 out]
                  n64 = Search 1D Array(1D array=w146, element=21) -> (index of element=w144:i32)  [unwired: 1 out]
                  n65 = case shown="-1" w144 {
                    tunnel: [string[] ["Add Filter Classes"] ("Strings [4]") string[] ["Add Classes"] ("Strings [4]")] -> w148
                    tunnel: [string[] ["Add Filter Directories"] ("Strings [4]") string[] ["Add Directories"] ("Strings [4]")] -> w147
                    tunnel: [string[] ["Add Filter Directories Recursively"] ("Strings [4]") string[] ["Add Directories Recursively"] ("Strings [4]")] -> w143
                    frame 0, Default {
                    }
                    frame -1 {
                    }
                  }
                  n66 = property on="AddClasses" class="Bool"("Strings [4]"=w148) -> ()  [unwired: 2 in, 2 out]
                  n67 = property on="AddDirs" class="Bool"("Strings [4]"=w147) -> ()  [unwired: 2 in, 2 out]
                  n68 = property on="AddDirsRec" class="Bool"("Strings [4]"=w143) -> ()  [unwired: 2 in, 2 out]
                }
                event "Help": Value Change {
                  n69 = event-data() -> ()  [unwired: 2 out]
                  n70 = case shown="True" "Help" {
                    tunnel: [ContextHelp_HelpTexts."None(Hide)" ("HelpText") ContextHelp_HelpTexts."UMLEditor reversedEngineering_Help" ("HelpText")] -> w157
                    frame False {
                    }
                    frame True {
                    }
                  }
                  n71 = call <resource>:"ContextHelp_HelpTexts.vi"("HelpText (enum or string)"=w157) -> ("HelpOut"=w158:T24)  [unwired: 18 out]
                  n72 = call <resource>:"ContextHelp_SendMessageToPopUp.vi"("PopUpMessage"=w158) -> ()  [unwired: 2 in, 17 out]
                }
                event Mouse Enter {
                  n73 = event-data() -> ("CtlRef"=w162:refnum<vi>)  [unwired: 1 out]
                  n74 = local read "Help"() -> (w161:bool)
                  n75 = call <resource>:"ContextHelp_CheckHelpForControl.vi"("Ctl Refnum"=w162, "Help"=w161) -> ()  [unwired: 1 in, 17 out]
                }
                event "ok": Value Change {
                  n76 = event-data() -> ()  [unwired: 6 out]
                  n77 = local read "files"() -> (w164:path[])
                  n78 = Empty Array?(array=w164) -> (empty?=w163:bool)
                }
                event "cancel": Value Change {
                  n79 = event-data() -> ()  [unwired: 6 out]
                }
                event "AddTopVIs", "AddClasses", "AddDirs", "AddDirsRec": Value Change {
                  w179 = ReversedEngineering_RecursiveSearchElements."Class" ("x")
                  w193 = UMLEditor_StoredPathes."LastSearchPath" ("UMLPathes")
                  n80 = event-data() -> ()  [unwired: 2 out]
                  n81 = Or(x="AddDirs", y="AddDirsRec") -> (x .or. y?=w171:bool)
                  n82 = Build Array("AddTopVIs", "AddClasses", w171) -> (w197:bool[])
                  n83 = Boolean Array To Number(Boolean array=w197) -> (number=w196:u32)
                  n84 = case shown="2" w196 {
                    tunnel: [T17."existing file" ("select mode (2)") T17."existing dir" ("select mode (2)") T17."existing file" ("select mode (2)")] -> w194
                    tunnel: ["*.lvclass" ("pattern") "*." ("pattern") "*.vi" ("pattern")] -> w191
                    tunnel: ["Select Class (llb or dir)" ("prompt") "Select directory" ("prompt") "Select TopVI" ("prompt")] -> w190
                    tunnel: "AddDirsRec" -> [_ w272 _]
                    tunnel: [_ w277 _] -> w183
                    tunnel: [ReversedEngineering_RecursiveSearchElements."Class" ("Enum") w273 ReversedEngineering_RecursiveSearchElements."TopVi" ("Enum")] -> w178
                    tunnel: ["Lv-Classes" ("pattern label") "Directory" ("pattern label") "TopVI" ("pattern label")] -> w187
                    frame 2 {
                    }
                    frame 4 {
                      n85 = Select(t=" (recursive)" ("pattern"), s=w272, f="") -> (s? t:f=w277:string)
                      n86 = Select(t=ReversedEngineering_RecursiveSearchElements."Dir(rec.)" ("Enum"), s=w272, f=ReversedEngineering_RecursiveSearchElements."Dir" ("Enum")) -> (s? t:f=w273:T2)
                    }
                    frame 1, Default {
                    }
                  }
                  n87 = call <resource>:"File_ApplicationPaths.vi"("PathName"=w193) -> ("Path Out"=w195:path)  [unwired: 3 in, 15 out]
                  n88 = call <vilib>:"compatFileDialog.vi"("pattern label"=w187, "button label"="Select", "prompt"=w190, "pattern"=w191, "select mode (2)"=w194, "start path"=w195) -> ("cancelled"=w168:bool, "path"=w176:path)  [unwired: 1 in, 3 out]
                  n89 = Not Equal?(x=w179, y=w178) -> (x != y?=w180:bool)
                  n90 = Equal?(x=w179, y=w178) -> (x = y?=w175:bool)
                  n91 = call <resource>:"Common_DoesClassExist.vi"("ClassPath"=w176, "ClassName"="No LLBs") -> ("ClassExists"=w186:bool)  [unwired: 17 out]
                  n92 = File/Directory Info(path=w176) -> (directory=w192:bool)  [unwired: 1 in, 6 out]
                  n93 = Strip Path(path=w176) -> (stripped path=w188:path)  [unwired: 1 out]
                  n94 = call <resource>:"Common_DoesClassExist.vi"("ClassPath"=w176) -> ("ClassExists"=w174:bool)  [unwired: 1 in, 17 out]
                  n95 = And(x=w180, y=w186) -> (x .and. y?=w185:bool)
                  n96 = Select(t=w176, s=w192, f=w188) -> (s? t:f=w189:path)
                  n97 = Compound Arithmetic op=AND(w175, invert w174) -> (w172:bool)
                  n98 = case shown="True" w185 {
                    tunnel: w178 -> [w201 _]
                    tunnel: [w201 ReversedEngineering_RecursiveSearchElements."Class" ("x")] -> w184
                    tunnel: w183 -> [w200 _]
                    tunnel: [w200 _] -> w182
                    frame False {
                    }
                    frame True {
                      n99 = One Button Dialog(message="This directory is identified as\na class-directory.") -> ()  [unwired: 2 out]
                    }
                  }
                  n100 = Or(x=w168, y=w172) -> (x .or. y?=w173:bool)
                  n101 = case shown="False" w173 {
                    tunnel: w193 -> [w224 _]
                    tunnel: w176 -> [w215 _]
                    tunnel: w182 -> [w218 _]
                    tunnel: w189 -> [w217 _]
                    tunnel: w184 -> [w204 _]
                    tunnel: w172 -> [_ w262]
                    tunnel: w168 -> [_ w261]
                    frame False {
                      n102 = local read "SearchElements"() -> (w208:T2[])
                      n103 = case shown="\"Class\"" w204 {
                        tunnel: [21 16 14 15] -> w206
                        frame "TopVi", Default {
                          n104 = property on="AddTopVIs" class="Bool"("Disabled"=u8 2) -> ()  [unwired: 2 in, 2 out]
                        }
                        frame "Class" {
                        }
                        frame "Dir" {
                        }
                        frame "Dir(rec.)" {
                        }
                      }
                      n105 = property on="Pathes" class="LstBox (strict)"() -> ("Item Names"=w223:string[], "Item Symbols"=w221:i32[])  [unwired: 2 in, 2 out]
                      n106 = local read "files"() -> (w216:path[])
                      n107 = Path To String(path=w215) -> (string=w219:string)
                      n108 = Concatenate Strings(w219, w218) -> (w213:string)
                      n109 = call <resource>:"File_ApplicationPaths.vi"("PathName"=w224, "Path In"=w217, "Method (Get Path)"=File_StoredPathesActions."Set Path") -> ()  [unwired: 1 in, 16 out]
                      n110 = String Length(string=w213) -> (length=w212:i32)
                      n111 = Subtract(x=w212, y=95) -> (x-y=w210:i32)
                      n112 = property on="Remove" class="Bool"("Disabled"=u8 0 ("t")) -> ()  [unwired: 2 in, 2 out]
                      n113 = case shown="1.." w210 {
                        selector: w210 -> [_ w259]
                        tunnel: w213 -> [w255 w260]
                        tunnel: [w255 w258] -> w209
                        frame 0, Default {
                        }
                        frame 1.. {
                          n114 = String Subset(string=w260, offset (0)=w259) -> (substring=w256:string)  [unwired: 1 out]
                          n115 = Concatenate Strings("..." ("string"), w256) -> (w258:string)
                        }
                      }
                      n116 = case shown="\"TopVi\"" w204 {
                        tunnel: w223 -> [w237 w241]
                        tunnel: [w236 w242] -> w222
                        tunnel: w221 -> [w235 w239]
                        tunnel: [w234 w238] -> w220
                        tunnel: w216 -> [w233 w244]
                        tunnel: w215 -> [w232 w246]
                        tunnel: [w231 w245] -> w214
                        tunnel: w209 -> [w230 w243]
                        tunnel: w208 -> [w229 w249]
                        tunnel: [w228 w247] -> w207
                        tunnel: w204 -> [w227 w248]
                        tunnel: w206 -> [w226 w240]
                        frame Default {
                          n117 = Build Array (concatenate)(w237, w230) -> (w236:string[])
                          n118 = Build Array (concatenate)(w235, w226) -> (w234:i32[])
                          n119 = Build Array (concatenate)(w229, w227) -> (w228:T2[])
                          n120 = Build Array (concatenate)(w233, w232) -> (w231:path[])
                        }
                        frame "TopVi" {
                          n121 = Build Array (concatenate)(w240, w239) -> (w238:i32[])
                          n122 = Build Array (concatenate)(w243, w241) -> (w242:string[])
                          n123 = Build Array (concatenate)(w246, w244) -> (w245:path[])
                          n124 = Build Array (concatenate)(w248, w249) -> (w247:T2[])
                        }
                      }
                      n125 = local write "SearchElements"(w207) -> ()
                      n126 = property on="Pathes" class="LstBox (strict)"("Item Names"=w222, "Item Symbols"=w220) -> ()  [unwired: 2 in, 2 out]
                      n127 = local write "files"(w214) -> ()
                    }
                    frame True {
                      n128 = case shown="True" w261 {
                        tunnel: w262 -> [w263 _]
                        frame False {
                          n129 = case shown="False" w263 {
                            frame False {
                            }
                            frame True {
                              n130 = One Button Dialog(message="This is not a class.\nSelect a class.") -> ()  [unwired: 2 out]
                            }
                          }
                        }
                        frame True {
                        }
                      }
                    }
                  }
                }
                event "ReverseCurrectProject": Value Change {
                  w292 = TRUE ("ExcludeDependencies")
                  n131 = event-data() -> ()  [unwired: 2 out]
                  n132 = call <resource>:"CommonVIs_UmlOpenVIRef.vi"() -> ("ProjectNameOut"=w291:string, "AppRefOut"=w288:refnum<vi>)  [unwired: 4 in, 6 out]
                  n133 = property class="App"(reference=w288) -> (error out=w289:errorcluster, "Project.TargetItem"=w290:refnum<vi>)  [unwired: 1 in, 1 out]
                  n134 = local write "Pathes"(i32[] [] ("Pathes")) -> ()
                  n135 = case shown="No Error" w289 {
                    tunnel: w291 -> [_ w313]
                    tunnel: [w306 w309] -> w287
                    tunnel: w290 -> [w306 _]
                    frame No Error {
                    }
                    frame Error {
                      n136 = call <resource>:"GDSProject_GetProjects.vi"("GetProjectRefByName"=w313) -> ("Project Refnum"=w308:refnum<vi>, "error out"=w312:errorcluster)  [unwired: 2 in, 15 out]
                      n137 = property class="Project"(reference=w308, error in=w312) -> (reference out=w307:refnum<vi>, "My Computer"=w311:refnum<vi>)  [unwired: 1 out]
                      n138 = To More Generic Class(target class=refnum<vi> refnum ("My Computer"), reference=w311) -> (generic class reference=w309:refnum<vi>)
                      n139 = Close Reference(reference=w307) -> ()  [unwired: 1 in, 1 out]
                    }
                  }
                  n140 = local read "SearchElements"() -> (w294:T2[])
                  n141 = property on="Pathes" class="LstBox (strict)"() -> ("Item Names"=w299:string[], "Item Symbols"=w298:i32[])  [unwired: 2 in, 2 out]
                  n142 = invoke class="ProjectItem" method="Get All Descendents"(reference=w287, "Type"="lvclass", "Exclude Dependencies"=w292, "ExcludeBuilds"=w292, "ExcludeTargets"=w292) -> (reference out=w302:refnum<vi>, error out=w303:errorcluster, "All Descendents"=w304:refnum<vi>[])  [unwired: 2 in, 4 out]
                  n143 = local read "files"() -> (w301:path[])
                  n144 = Close Reference(reference=w302, error in (no error)=w303) -> ()  [unwired: 1 out]
                  n145 = for {
                    tunnel: w304 -> [w328] mode=indexing
                    shift-right: [w320] -> w300
                    shift-left: w301 -> [w319]
                    shift-right: [w322] -> w296
                    shift-left: w298 -> [w324]
                    shift-right: [w321] -> w297
                    shift-left: w299 -> [w326]
                    shift-right: [w316] -> w293
                    shift-left: w294 -> [w315]
                    n146 = property class="ProjectItem"(reference=w328) -> (reference out=w327:refnum<vi>, "Path"=w318:path)  [unwired: 1 in, 1 out]
                    n147 = call <vilib>:"Get File Extension.vi"("file"=w318) -> ("filename without extension"=w325:string)  [unwired: 1 in, 9 out]
                    n148 = Search 1D Array(1D array=w319, element=w318) -> (index of element=w317:i32)  [unwired: 1 out]
                    n149 = Close Reference(reference=w327) -> ()  [unwired: 1 in, 1 out]
                    n150 = case shown="0, Default" w317 {
                      tunnel: w319 -> [w330 w344]
                      tunnel: w318 -> [_ w343]
                      tunnel: w326 -> [w332 w342]
                      tunnel: w325 -> [_ w341]
                      tunnel: w324 -> [w331 w340]
                      tunnel: 16 -> [_ w339]
                      tunnel: [w331 w338] -> w322
                      tunnel: [w332 w337] -> w321
                      tunnel: [w330 w336] -> w320
                      tunnel: [w329 w335] -> w316
                      tunnel: w315 -> [w329 w334]
                      tunnel: ReversedEngineering_RecursiveSearchElements."Class" ("x") -> [_ w333]
                      frame 0, Default {
                      }
                      frame -1 {
                        n151 = Build Array (concatenate)(w344, w343) -> (w336:path[])
                        n152 = Build Array (concatenate)(w334, w333) -> (w335:T2[])
                        n153 = Build Array (concatenate)(w342, w341) -> (w337:string[])
                        n154 = Build Array (concatenate)(w340, w339) -> (w338:i32[])
                      }
                    }
                  }
                  n155 = local write "ReverseCurrectProject"(FALSE ("ReverseCurrectProject")) -> ()
                  n156 = property on="Pathes" class="LstBox (strict)"("Item Names"=w297, "Item Symbols"=w296) -> ()  [unwired: 2 in, 2 out]
                  n157 = local write "SearchElements"(w293) -> ()
                  n158 = local write "files"(w300) -> ()
                }
                event "ClearList": Value Change {
                  w345 = T2[] [] items=["TopVi", "Class", "Dir", "Dir(rec.)"] ("SearchElements")
                  n159 = event-data() -> ()  [unwired: 2 out]
                  n160 = local write "SearchElements"(w345) -> ()
                  n161 = property on="Remove" class="Bool"("Disabled"=u8 2) -> ()  [unwired: 2 in, 2 out]
                  n162 = property on="Pathes" class="LstBox (strict)"("Item Names"=string[] [], "Item Symbols"=i32[] []) -> ()  [unwired: 2 in, 2 out]
                  n163 = local write "files"(path[] [] ("files")) -> ()
                }
                event "Remove": Value Change {
                  n164 = event-data() -> ()  [unwired: 2 out]
                  n165 = local read "files"() -> (w371:path[])
                  n166 = local read "Pathes"() -> (w360:i32[])
                  n167 = Array Size(array=w371) -> (size(s)=w370:i32)
                  n168 = Decrement(x=w370) -> (x-1=w369:i32)
                  n169 = Empty Array?(array=w360) -> (empty?=w359:bool)
                  n170 = Build Array(w369) -> (w361:i32[])
                  n171 = local read "SearchElements"() -> (w373:T2[])
                  n172 = property on="Pathes" class="LstBox (strict)"() -> ("Item Names"=w380:string[], "Item Symbols"=w379:i32[])  [unwired: 2 in, 2 out]
                  n173 = Select(t=w361, s=w359, f=w360) -> (s? t:f=w372:i32[])
                  n174 = Sort 1D Array(array=w372) -> (sorted array=w358:i32[])
                  n175 = Reverse 1D Array(array=w358) -> (reversed array=w357:i32[])
                  n176 = for {
                    tunnel: w357 -> [w383] mode=indexing
                    shift-right: [w386] -> w377
                    shift-left: w371 -> [w382]
                    shift-right: [w387] -> w378
                    shift-left: w379 -> [w388]
                    shift-right: [w385] -> w356
                    shift-left: w380 -> [w389]
                    shift-right: [w381] -> w368
                    shift-left: w373 -> [w384]
                    n177 = Delete From Array(array=w382, index=w383) -> (array with subset deleted=w386:path[])  [unwired: 1 in, 1 out]
                    n178 = Delete From Array(array=w389, index=w383) -> (array with subset deleted=w385:string[])  [unwired: 1 in, 1 out]
                    n179 = Delete From Array(array=w388, index=w383) -> (array with subset deleted=w387:i32[])  [unwired: 1 in, 1 out]
                    n180 = Delete From Array(array=w384, index=w383) -> (array with subset deleted=w381:T2[])  [unwired: 1 in, 1 out]
                  }
                  n181 = Array Size(array=w356) -> (size(s)=w355:i32)
                  n182 = Equal?(x=ReversedEngineering_RecursiveSearchElements."TopVi" ("deleted portion"), y=w368) -> (x = y?=w366:bool[])
                  n183 = Empty Array?(array=w356) -> (empty?=w354:bool)
                  n184 = Decrement(x=w355) -> (x-1=w353:i32)
                  n185 = Or Array Elements(Boolean array=w366) -> (logical OR=w365:bool)
                  n186 = Build Array(w353) -> (w352:i32[])
                  n187 = Select(t=u8 2 ("Disabled"), s=w365, f=u8 0) -> (s? t:f=w363:u8)
                  n188 = local write "SearchElements"(w368) -> ()
                  n189 = Select(t=u8 0, s=w354, f=u8 2 ("Disabled")) -> (s? t:f=w375:u8)
                  n190 = Select(t=i32[] [], s=w354, f=w352) -> (s? t:f=w351:i32[])
                  n191 = property on="AddTopVIs" class="Bool"("Disabled"=w363) -> ()  [unwired: 2 in, 2 out]
                  n192 = property on="Pathes" class="LstBox (strict)"("Item Names"=w356, "Item Symbols"=w378) -> ()  [unwired: 2 in, 2 out]
                  n193 = local write "files"(w377) -> ()
                  n194 = property on="Remove" class="Bool"("Disabled"=w375) -> ()  [unwired: 2 in, 2 out]
                  n195 = local write "Pathes"(w351) -> ()
                }
                event "Pathes": Value Change {
                  n196 = event-data() -> ()  [unwired: 2 out]
                  n197 = Empty Array?(array="Pathes") -> (empty?=w393:bool)
                  n198 = Select(t=T18."Disabled and Grayed Out" ("Disabled"), s=w393, f=T18."Enabled" ("Disabled")) -> (s? t:f=w390:T18)
                  n199 = property on="Remove" class="Bool"("Disabled"=w390) -> ()  [unwired: 2 in, 2 out]
                }
              }
            }
            n200 = call <resource>:"CommonVIs_CloseControlRefs.vi"("Event Registration Refnum"=w129, "ControlRefs"=w128) -> ()  [unwired: 1 in, 17 out]
            n201 = Bundle By Name(cluster=w133, "cancel"=w131) -> (w132:T3)
            n202 = Select(t="Exit", s=w131, f="GetReverserdInfo") -> (s? t:f=w135:string)
          }
          frame "AnalyseClass" {
            n203 = call <vilib>:"Get File Extension.vi"("file"=w398) -> ("filename without extension"=w397:string)  [unwired: 1 in, 9 out]
            n204 = Build Array(w398) -> (w400:path[])
            n205 = Build Array(w397) -> (w402:string[])
            n206 = Build Array(16) -> (w401:i32[])
            n207 = local write "HideSubAss"(TRUE ("HideSubAss")) -> ()
            n208 = local write "OnlyInheritance"(FALSE ("OnlyInheritance")) -> ()
            n209 = property on="Pathes" class="LstBox (strict)"("Item Names"=w402, "Item Symbols"=w401) -> ()  [unwired: 2 in, 2 out]
            n210 = local write "files"(w400) -> ()
          }
          frame "GetReverserdInfo" {
            w410 = "Reverse Engineering" ("Title/StatusText")
            n211 = property on="Pathes" class="LstBox (strict)"() -> ("Item Names"=w408:string[])  [unwired: 2 in, 2 out]
            n212 = Array Size(array=w408) -> (size(s)=w407:i32)
            n213 = Format Into String(format string=" %d classes", initial string=w410, w407) -> (resulting string=w406:string)  [unwired: 1 in, 1 out]
            n214 = call <resource>:"CommonVIs_TimingLogger2.vi"("error in (no error)"=w433, "Name"=w406) -> ("error out"=w411:errorcluster)  [unwired: 9 in]
            n215 = Not(x=w420) -> (.not. x?=w419:bool)
            n216 = call <resource>:"UMLEditor ControlBusyDialog.vi"("Title/StatusText"=w410, "error in (no error)"=w411, "Action(SendStatusMessage)"=UMLEditor_BusyDialogAction."Open(i)" ("Action")) -> ("error out"=w431:errorcluster)  [unwired: 1 in, 15 out]
            n217 = local read "OnlyInheritance"() -> (w441:bool)
            n218 = stacked-sequence {
              tunnel: [w451] -> w432
              tunnel: w431 -> [w451]
              frame #0 {
                n219 = Wait (ms)(milliseconds to wait=u32 5) -> ()  [unwired: 1 out]
              }
            }
            n220 = local read "files"() -> (w442:path[])
            n221 = local read "SearchElements"() -> (w435:T2[])
            n222 = Select(t="RemoveNodes?" ("y"), s=w441, f="CreateNodes" ("y")) -> (s? t:f=w438:string)
            n223 = call <resource>:"ReversedEngineering GetCompleteDependencyInfo.vi"("path"=w442, "SearchElements"=w435, "error in (no error)"=w432, "Only Create this class and its dependencis"=w419, "SyncOption"="SyncOption", "CreateApplicationNode"="CreateApplication") -> ("classInfos"=w417:T4[], "TypeDefs"=w444:T11[], "Cancelled"=w424:bool, "error out"=w430:errorcluster)  [unwired: 2 in, 8 out]
            n224 = Select(t=w444, s="CreateTypes", f=T11[] []) -> (s? t:f=w418:T11[])
            n225 = Select(t="Hide SubClass ass. to classes that BaseClass already Assosiactes to" ("y"), s="HideSubAss", f=w438) -> (s? t:f=w422:string)
            n226 = Empty Array?(array=w417) -> (empty?=w416:bool)
            n227 = Empty Array?(array=w418) -> (empty?=w413:bool)
            n228 = Bundle By Name(cluster=w448, "cancel"=w424, "classInfos"=w417, "TypeDefs"=w418) -> (w449:T3)
            n229 = And(x=w416, y=w413) -> (x .and. y?=w414:bool)
            n230 = call <resource>:"UMLEditor ControlBusyDialog.vi"("Title/StatusText"="Removing VIs from memory", "error in (no error)"=w430) -> ("error out"=w429:errorcluster)  [unwired: 2 in, 15 out]
            n231 = Or(x=w424, y=w414) -> (x .or. y?=w415:bool)
            n232 = call <resource>:"ReversedEngineering ViCachMemory.vi"("RemoveAllCachedViRefs(False)"=TRUE, "error in (no error)"=w429) -> ("error out"=w427:errorcluster)  [unwired: 2 in, 15 out]
            n233 = Select(t="Exit", s=w415, f=w422) -> (s? t:f=w421:string)
            n234 = call <resource>:"UMLEditor ControlBusyDialog.vi"("Title/StatusText"="VIs removed", "error in (no error)"=w427) -> ("error out"=w426:errorcluster)  [unwired: 2 in, 15 out]
          }
          frame "ReadXMI-File" {
            n235 = call <resource>:"UMLEditor_ReadXmiFile.vi"("XmiFilePath"=w454, "error in (no error)"=w460) -> ("classInfos"=w458:T4[], "TypeDefs"=w457:T11[], "Positions"=w452:cluster{"X":i32, "Y":i32}[], "error out"=w456:errorcluster)  [unwired: 14 in]
            n236 = Bundle By Name(cluster=w459, "classInfos"=w458, "TypeDefs"=w457, "Positions"=w452) -> (w455:T3)
          }
          frame "Hide SubClass ass. to classes that BaseClass already Assosiactes to" {
            n237 = Unbundle By Name(w469) -> ("classInfos"=w470:T4[])
            n238 = Unbundle By Name(w469) -> ("classInfos"=w467:T4[])
            n239 = for {
              tunnel: w467 -> [w473] mode=indexing
              tunnel: [w472] -> w468 mode=indexing
              n240 = Unbundle By Name(w473) -> ("classPath"=w472:path)
            }
            n241 = for {
              tunnel: w470 -> [w477] mode=indexing
              tunnel: w468 -> [w475]
              tunnel: w467 -> [w478]
              tunnel: [w476] -> w466 mode=indexing
              n242 = Unbundle By Name(w477) -> ("inherits"=w479:bool, "baseClasses"=w474:path[])
              n243 = case shown="True" w479 {
                tunnel: w478 -> [_ w485]
                tunnel: w477 -> [w480 w484]
                tunnel: [w480 w483] -> w476
                tunnel: w475 -> [_ w482]
                tunnel: w474 -> [_ w481]
                frame False {
                }
                frame True {
                  n244 = for {
                    tunnel: w485 -> [w499]
                    shift-right: [w489] -> w483
                    shift-left: w484 -> [w490]
                    tunnel: w482 -> [w488]
                    tunnel: w481 -> [w487] mode=indexing
                    n245 = Search 1D Array(1D array=w488, element=w487) -> (index of element=w486:i32)  [unwired: 1 out]
                    n246 = Index Array(array=w499, index=w486) -> (element=w498:T4)
                    n247 = Unbundle By Name(w490) -> ("depClasses"=w494:path[])
                    n248 = Unbundle By Name(w498) -> ("compAggClasses"=w497:path[], "aggClasses"=w496:path[], "depClasses"=w495:path[])
                    n249 = Build Array (concatenate)(w497, w496, w495) -> (w493:path[])
                    n250 = for {
                      tunnel: w494 -> [w500] mode=indexing
                      tunnel: w493 -> [w504]
                      shift-right: [w502] -> w491
                      shift-left: path[] [] -> [w501]
                      n251 = Search 1D Array(1D array=w504, element=w500) -> (index of element=w503:i32)  [unwired: 1 out]
                      n252 = case shown="0, Default" w503 {
                        tunnel: [w505 w508] -> w502
                        tunnel: w501 -> [w505 w507]
                        tunnel: w500 -> [_ w506]
                        frame 0, Default {
                        }
                        frame -1 {
                          n253 = Build Array (concatenate)(w507, w506) -> (w508:path[])
                        }
                      }
                    }
                    n254 = Bundle By Name(cluster=w490, "depClasses"=w491) -> (w489:T4)
                  }
                }
              }
            }
            n255 = Bundle By Name(cluster=w469, "classInfos"=w466) -> (w471:T3)
            n256 = Select(t="RemoveNodes?" ("y"), s="OnlyInheritance", f="CreateNodes" ("y")) -> (s? t:f=w461:string)
          }
          frame "RemoveNodes?" {
            n257 = Unbundle By Name(w511) -> ("classInfos"=w512:T4[])
            n258 = Unbundle By Name(w511) -> ("classInfos"=w519:T4[])
            n259 = for {
              tunnel: w512 -> [w544] mode=indexing
              tunnel: [w543] -> w513 mode=indexing
              n260 = Unbundle By Name(w544) -> ("classPath"=w543:path)
            }
            n261 = Index Array(array=w519) -> (element=w517:T4)  [unwired: 1 in]
            n262 = Initialize Array(w517) -> (w518:T4[])  [unwired: 1 out]
            n263 = for {
              tunnel: w519 -> [w550] mode=indexing
              shift-right: [w548] -> w514
              shift-left: w518 -> [w549]
              shift-right: [w545] -> w515
              shift-left: path[] [] -> [w547]
              n264 = Unbundle By Name(w550) -> ("inherits"=w551:bool, "baseClasses"=w546:path[])
              n265 = case shown="True" w551 {
                tunnel: w550 -> [_ w560]
                tunnel: w549 -> [w552 w561]
                tunnel: [w552 w555] -> w548
                tunnel: w547 -> [w553 w554]
                tunnel: w546 -> [_ w559]
                tunnel: [w553 w556] -> w545
                frame False {
                }
                frame True {
                  n266 = Build Array (concatenate)(w561, w560) -> (w555:T4[])
                  n267 = Index Array(array=w559) -> (element=w557:path)  [unwired: 1 in]
                  n268 = Search 1D Array(1D array=w554, element=w557) -> (index of element=w558:i32)  [unwired: 1 out]
                  n269 = case shown="-1" w558 {
                    tunnel: w554 -> [w562 w565]
                    tunnel: w557 -> [_ w564]
                    tunnel: [w562 w563] -> w556
                    frame 0, Default {
                    }
                    frame -1 {
                      n270 = Build Array (concatenate)(w565, w564) -> (w563:path[])
                    }
                  }
                }
              }
            }
            n271 = for {
              tunnel: w515 -> [w524] mode=indexing
              shift-right: [w530] -> w510
              shift-left: w514 -> [w522]
              tunnel: w513 -> [w529]
              tunnel: w512 -> [w528]
              n272 = for {
                N -> [w540]
                tunnel: w522 -> [w542] mode=indexing
                tunnel: [w541] -> w525 mode=indexing
                tunnel: [w540] -> _ mode=indexing
                n273 = Unbundle By Name(w542) -> ("classPath"=w541:path)
              }
              n274 = Search 1D Array(1D array=w525, element=w524) -> (index of element=w523:i32)  [unwired: 1 out]
              n275 = Search 1D Array(1D array=w529, element=w524) -> (index of element=w526:i32)  [unwired: 1 out]
              n276 = Index Array(array=w528, index=w526) -> (element=w527:T4)
              n277 = case shown="0, Default" w523 {
                tunnel: w522 -> [w531 w535]
                tunnel: [w531 w534] -> w530
                tunnel: w527 -> [_ w533]
                tunnel: w526 -> [_ w532]
                frame 0, Default {
                }
                frame -1 {
                  n278 = case shown="0, Default" w532 {
                    tunnel: w535 -> [w538 w539]
                    tunnel: w533 -> [w537 _]
                    tunnel: [w536 w539] -> w534
                    frame 0, Default {
                      n279 = Build Array (concatenate)(w538, w537) -> (w536:T4[])
                    }
                    frame -1 {
                    }
                  }
                }
              }
            }
            n280 = Bundle By Name(cluster=w511, "classInfos"=w510) -> (w509:T3)
          }
          frame "CreateNodes" {
            n281 = Unbundle By Name(w578) -> ("classInfos"=w573:T4[], "Positions"=w571:cluster{"X":i32, "Y":i32}[])
            n282 = Array Size(array=w573) -> (size(s)=w572:i32)
            n283 = for {
              N: w572 -> [w598]
              shift-right: [w601] -> w567
              shift-left: w568 -> [w614]
              tunnel: w573 -> [w581] mode=indexing
              tunnel: [w593] -> w576 mode=indexing
              shift-right: [w603] -> w574
              shift-left: i32[] [] -> [w604]
              tunnel: w571 -> [w587]
              shift-right: [w588] -> w569
              shift-left: i32[] [] -> [w589]
              i -> [w586]
              n284 = Unbundle By Name(w581) -> ("Interface"=w580:bool)
              n285 = call <resource>:"ReversedEngineering ConvertAttributesAndMethodsToString.vi"("classInfo"=w581, "error in (no error)"=w614) -> ("StereoType"=w602:string, "className"=w616:string, "attributes"=w612:string, "methods"=w608:string, "ClassPath"=w596:path, "error out"=w615:errorcluster)  [unwired: 12 out]
              n286 = Array Size(array=w587) -> (size(s)=w584:i32)
              n287 = case shown="True" w580 {
                tunnel: [w624 w627] -> w621
                tunnel: [w623 w626] -> w620
                tunnel: w615 -> [w622 w625]
                frame True {
                  n288 = call <resource>:"InterfaceNode_Create.vi"("error in (no error)"=w622) -> ("reference out"=w624:refnum<class "InterfaceNode.lvclass">, "error out"=w623:errorcluster)  [unwired: 17 in]
                }
                frame False {
                  n289 = call <resource>:"ClassNode_Create.vi"("error in (no error)"=w625) -> ("reference out"=w627:refnum<class "ClassNode.lvclass">, "error out"=w626:errorcluster)  [unwired: 1 in, 16 out]
                }
              }
              n290 = Index Array(array=w587, index=w586) -> (element=w582:cluster{"X":i32, "Y":i32})
              n291 = Increment(x=w586) -> (x+1=w585:i32)
              n292 = Greater Or Equal?(x=w585, y=w584) -> (x >= y?=w583:bool)
              n293 = call-dynamic "ExternalSetParam.vi"("reference"=w621, "setParameter"=ExternalSetTypes."Name", "string"=w616, "error in (no error)"=w620) -> ("reference out"=w618:refnum<class "ClassNode.lvclass">, "error out"=w617:errorcluster)  [unwired: 14 in]
              n294 = case shown="True" w583 {
                tunnel: [w630 -1 ("X")] -> w591
                tunnel: [w629 _] -> w590
                tunnel: w582 -> [w628 _]
                frame False {
                  n295 = Unbundle(w628) -> ("X"=w630:i32, "Y"=w629:i32)
                }
                frame True {
                }
              }
              n296 = case shown="\"APPLICATION\"" w602 {
                tunnel: w604 -> [w644 w647]
                tunnel: w586 -> [_ w646]
                tunnel: [w644 w645] -> w603
                frame "False", Default {
                }
                frame "APPLICATION" {
                  n297 = Build Array (concatenate)(w647, w646) -> (w645:i32[])
                }
              }
              n298 = call-dynamic "ExternalSetParam.vi"("reference"=w618, "setParameter"=ExternalSetTypes."Attributes", "string"=w612, "error in (no error)"=w617) -> ("reference out"=w610:refnum<class "ClassNode.lvclass">, "error out"=w611:errorcluster)  [unwired: 14 in]
              n299 = Increment(x=w586) -> (x+1=w597:i32)
              n300 = call-dynamic "ExternalSetParam.vi"("reference"=w610, "setParameter"=ExternalSetTypes."Methods", "string"=w608, "error in (no error)"=w611) -> ("reference out"=w606:refnum<class "ClassNode.lvclass">, "error out"=w607:errorcluster)  [unwired: 14 in]
              n301 = call-dynamic "ExternalSetParam.vi"("reference"=w606, "setParameter"=ExternalSetTypes."ClassPath", "error in (no error)"=w607, "ClassPath"=w596) -> ("reference out"=w592:refnum<class "ClassNode.lvclass">, "error out"=w595:errorcluster)  [unwired: 14 in]
              n302 = case shown="0, Default" w591 {
                selector: w591 -> [w636 _]
                tunnel: w595 -> [w640 w642]
                tunnel: [w639 w642] -> w594
                tunnel: [w638 w643] -> w593
                tunnel: w592 -> [w637 w643]
                tunnel: w590 -> [w635 _]
                tunnel: w589 -> [w634 w641]
                tunnel: w586 -> [w633 _]
                tunnel: [w632 w641] -> w588
                frame 0, Default {
                  n303 = call <resource>:"setPosition.vi"("reference"=w637, "x"=w636, "y"=w635, "error in (no error)"=w640) -> ("reference out"=w638:refnum<class "ClassNode.lvclass">, "error out"=w639:errorcluster)  [unwired: 1 in, 13 out]
                  n304 = Build Array (concatenate)(w634, w633) -> (w632:i32[])
                }
                frame -1 {
                }
              }
              n305 = Format Into String(format string="Creating classes %d of %d", w597, w598) -> (resulting string=w600:string)  [unwired: 2 in, 1 out]
              n306 = call <resource>:"UMLEditor ControlBusyDialog.vi"("Title/StatusText"=w600, "error in (no error)"=w594) -> ("error out"=w601:errorcluster)  [unwired: 2 in, 15 out]
            }
            "ApplicationNodes" <- w574
            n307 = Bundle By Name(cluster=w578, "nodes"=w576, "nodesDone"=w569) -> (w577:T3)
            n308 = call <resource>:"CommonVIs_TimingLogger2.vi"("error in (no error)"=w567) -> ("error out"=w566:errorcluster)  [unwired: 10 in]
          }
          frame "RemoveDubbleTypeDefs" {
            n309 = Unbundle By Name(w653) -> ("TypeDefs"=w654:T11[])
            n310 = for {
              tunnel: w654 -> [w666] mode=indexing
              shift-right: [w665] -> w650
              shift-left: T11[] [] -> [w667]
              tunnel: string[] ["ClassAttributes$", "ObjectAttributes$", "ObjectReference$"] -> [w656]
              n311 = Unbundle By Name(w666) -> ("TypeDefPath"=w663:path, "TypeDefName"=w662:string)
              n312 = for {
                tunnel: w667 -> [w677] mode=indexing
                tunnel: [w676] -> w664 mode=indexing
                n313 = Unbundle By Name(w677) -> ("TypeDefPath"=w676:path)
              }
              n314 = for {
                tunnel: w662 -> [w671]
                tunnel: [w669] -> w658 mode=indexing
                tunnel: w656 -> [w668] mode=indexing
                n315 = Match Pattern(string=w671, regular expression=w668) -> (offset past match=w670:i32)  [unwired: 4 out]
                n316 = Greater Or Equal To 0?(x=w670) -> (x >= 0?=w669:bool)
              }
              n317 = Or Array Elements(Boolean array=w658) -> (logical OR=w657:bool)
              n318 = Search 1D Array(1D array=w664, element=w663) -> (index of element=w661:i32)  [unwired: 1 out]
              n319 = Greater Or Equal To 0?(x=w661) -> (x >= 0?=w659:bool)
              n320 = Or(x=w659, y=w657) -> (x .or. y?=w660:bool)
              n321 = case shown="True" w660 {
                tunnel: w667 -> [w672 w675]
                tunnel: w666 -> [_ w674]
                tunnel: [w672 w673] -> w665
                frame True {
                }
                frame False {
                  n322 = Build Array (concatenate)(w675, w674) -> (w673:T11[])
                }
              }
            }
            n323 = Bundle By Name(cluster=w653, "TypeDefs"=w650) -> (w652:T3)
          }
          frame "CreateTypeDefsNodes" {
            n324 = Unbundle By Name(w683) -> ("TypeDefs"=w685:T11[])
            n325 = for {
              shift-right: [w695] -> w679
              shift-left: w686 -> [w713]
              tunnel: w685 -> [w692] mode=indexing
              tunnel: [w694] -> w680 mode=indexing
              n326 = Unbundle By Name(w692) -> ("TypeDefAttribInfo"=w707:T6[], "TypeDefName"=w711:string, "TypeDefPath"=w691:path)
              n327 = call <resource>:"ReversedEngineering CheckCtlStereoType.vi"("TypeDefPath"=w691) -> ("ClassDesc"=w689:string)
              n328 = Equal?(x=w689, y="<<ENUM>>" ("ClassDesc")) -> (x = y?=w688:bool)
              n329 = for {
                tunnel: [w722] -> w706 mode=indexing
                tunnel: w707 -> [w721] mode=indexing
                tunnel: w688 -> [w718]
                n330 = Unbundle By Name(w721) -> ("name"=w723:string, "type"=w727:T7, "dimension"=w725:i32, "typeName"=w726:string)
                n331 = call <resource>:"ReversedEngineering AttributesTypeToString.vi"("AttributeDataType"=w727, "name"=w726) -> ("string"=w720:string)  [unwired: 17 out]
                n332 = case shown="\"\"" w720 {
                  tunnel: [" : " _] -> w719
                  frame Default {
                  }
                  frame "" {
                  }
                }
                n333 = for {
                  N: w725 -> [_]
                  tunnel: ["[]"] -> w724 mode=indexing
                }
                n334 = case shown="True" w718 {
                  tunnel: w724 -> [w732 _]
                  tunnel: w723 -> [w731 w733]
                  tunnel: [w730 w733] -> w722
                  tunnel: w720 -> [w729 _]
                  tunnel: w719 -> [w728 _]
                  frame False {
                    n335 = Concatenate Strings(w731, w732, w728, w729) -> (w730:string)
                  }
                  frame True {
                  }
                }
              }
              n336 = Format Into String(format string="%s\n%s", w689, w711) -> (resulting string=w710:string)  [unwired: 2 in, 1 out]
              n337 = call <resource>:"ClassNode_Create.vi"("error in (no error)"=w713) -> ("reference out"=w717:refnum<class "ClassNode.lvclass">, "error out"=w716:errorcluster)  [unwired: 1 in, 16 out]
              n338 = call-dynamic "ExternalSetParam.vi"("reference"=w717, "setParameter"=ExternalSetTypes."Name", "string"=w710, "error in (no error)"=w716) -> ("reference out"=w702:refnum<class "ClassNode.lvclass">, "error out"=w700:errorcluster)  [unwired: 14 in]
              n339 = Array To Spreadsheet String(delimiter (Tab)="\n", array=w706, 3:"%s" ("format string")) -> (spreadsheet string=w705:string)
              n340 = call-dynamic "ExternalSetParam.vi"("reference"=w702, "setParameter"=ExternalSetTypes."ShowMethods", "Boolean"=FALSE, "error in (no error)"=w700) -> ("reference out"=w701:refnum<class "ClassNode.lvclass">, "error out"=w699:errorcluster)  [unwired: 14 in]
              n341 = call <vilib>:"Trim Whitespace.vi"("string"=w705) -> ("trimmed string"=w704:string)  [unwired: 1 in]
              n342 = call-dynamic "ExternalSetParam.vi"("reference"=w701, "setParameter"=ExternalSetTypes."Attributes", "string"=w704, "error in (no error)"=w699) -> ("reference out"=w693:refnum<class "ClassNode.lvclass">, "error out"=w696:errorcluster)  [unwired: 14 in]
              n343 = call-dynamic "ExternalSetParam.vi"("reference"=w693, "setParameter"=ExternalSetTypes."ClassPath", "error in (no error)"=w696, "ClassPath"=w691) -> ("reference out"=w694:refnum<class "ClassNode.lvclass">, "error out"=w695:errorcluster)  [unwired: 14 in]
            }
            n344 = Unbundle By Name(w683) -> ("nodes"=w682:refnum<class "ClassNode.lvclass">[])
            n345 = Build Array (concatenate)(w682, w680) -> (w681:refnum<class "ClassNode.lvclass">[])
            n346 = Bundle By Name(cluster=w683, "nodes"=w681) -> (w684:T3)
            n347 = call <resource>:"CommonVIs_TimingLogger2.vi"("error in (no error)"=w679) -> ("error out"=w678:errorcluster)  [unwired: 10 in]
          }
          frame "CreateEdges" {
            w739 = TRUE  # Show Multiplicity
            n348 = Unbundle By Name(w741) -> ("nodes"=w742:refnum<class "ClassNode.lvclass">[], "classInfos"=w743:T4[])
            n349 = for {
              shift-right: [w747] -> w738
              shift-left: w744 -> [w752]
              tunnel: w743 -> [w748] mode=indexing
              tunnel: w742 -> [w750] mode=indexing
              tunnel: w742 -> [w749]
              tunnel: w739 -> [w751]
              tunnel: [w746] -> w736 mode=concatenating
              n350 = call <resource>:"ReversedEngineering CreateEdges.vi"("NodeRef"=w750, "AllNodes"=w749, "NodeClassInfo"=w748, "error in (no error)"=w752, "Show Multiplicity"=w751) -> ("EdgesCreated"=w746:refnum<class "AbstractEdge.lvclass">[], "error out"=w747:errorcluster)  [unwired: 1 in, 12 out]
            }
            n351 = Bundle By Name(cluster=w741, "edges"=w736) -> (w740:T3)
            n352 = call <resource>:"CommonVIs_TimingLogger2.vi"("error in (no error)"=w738) -> ("error out"=w737:errorcluster)  [unwired: 10 in]
          }
          frame "CreateTypeDefEdgesFromClasses" {
            n353 = Unbundle By Name(w763) -> ("edges"=w762:refnum<class "AbstractEdge.lvclass">[], "TypeDefs"=w757:T11[])
            n354 = Unbundle By Name(w763) -> ("nodes"=w760:refnum<class "ClassNode.lvclass">[], "classInfos"=w761:T4[])
            n355 = Array Size(array=w761) -> (size(s)=w759:i32)
            n356 = Array Subset(array=w760, index=w759) -> (w758:refnum<class "ClassNode.lvclass">[])  [unwired: 1 in]
            n357 = for {
              shift-right: [w770] -> w754
              shift-left: w766 -> [w769]
              tunnel: w758 -> [w768] mode=indexing
              tunnel: w761 -> [w774]
              tunnel: w760 -> [w767]
              shift-right: [w771] -> w764
              shift-left: w762 -> [w772]
              tunnel: w757 -> [w775] mode=indexing
              tunnel: string[] [] -> [_]
              # "Association"
              n358 = Unbundle By Name(w775) -> ("TypeDefPath"=w773:path)
              n359 = for {
                tunnel: w774 -> [w781] mode=indexing
                tunnel: w773 -> [w789]
                shift-right: [w787] -> w771
                shift-left: w772 -> [w788]
                shift-right: [w782] -> w770
                shift-left: w769 -> [w785]
                tunnel: [w785] -> _ mode=indexing
                tunnel: w768 -> [w784]
                tunnel: w767 -> [w783] mode=indexing
                n360 = Unbundle By Name(w781) -> ("objectAttrib"=w792:T6[], "classAttrib"=w791:T6[])
                n361 = Unbundle By Name(w781) -> ("DependencyDetails"=w780:T8[])
                n362 = Build Array (concatenate)(w792, w791) -> (w790:T6[])
                n363 = for {
                  tunnel: w790 -> [w821] mode=indexing
                  tunnel: [w820] -> w779 mode=indexing
                  n364 = Unbundle By Name(w821) -> ("typePath"=w820:path)
                }
                n365 = for {
                  tunnel: w780 -> [w796] mode=indexing
                  shift-right: [w795] -> w777
                  shift-left: path[] [] -> [w793]
                  n366 = Unbundle By Name(w796) -> ("Dependent_VIs/Ctls"=w794:path[])
                  n367 = Build Array (concatenate)(w793, w794) -> (w795:path[])
                }
                n368 = Build Array (concatenate)(w777, w779) -> (w778:path[])
                n369 = Search 1D Array(1D array=w778, element=w789) -> (index of element=w786:i32)  [unwired: 1 out]
                n370 = case shown="0, Default" w786 {
                  tunnel: w784 -> [w817 _]
                  tunnel: [w799 w818] -> w782
                  tunnel: w783 -> [w797 _]
                  tunnel: w788 -> [w816 w819]
                  tunnel: [w815 w819] -> w787
                  tunnel: w785 -> [w798 w818]
                  frame 0, Default {
                    n371 = call <resource>:"ClassRelationshipEdge_Create.vi"("error in (no error)"=w798) -> ("reference out"=w814:refnum<class "ClassRelationshipEdge.lvclass">, "error out"=w813:errorcluster)  [unwired: 1 in, 16 out]
                    n372 = call-dynamic "externalSetParam.vi"("reference"=w814, "node"=w817, "error in (no error)"=w813, "setParam"=ExternaSetParamType."EndNode") -> ("reference out"=w811:refnum<class "ClassRelationshipEdge.lvclass">, "error out"=w810:errorcluster)  [unwired: 14 in]
                    n373 = call-dynamic "externalSetParam.vi"("reference"=w811, "node"=w797, "error in (no error)"=w810, "setParam"=ExternaSetParamType."StartNode") -> ("reference out"=w809:refnum<class "ClassRelationshipEdge.lvclass">, "error out"=w808:errorcluster)  [unwired: 14 in]
                    n374 = call-dynamic "externalSetParam.vi"("reference"=w809, "arrowHead"=ArrowHeadType."V", "error in (no error)"=w808, "setParam"=ExternaSetParamType."EndArrow") -> ("reference out"=w807:refnum<class "ClassRelationshipEdge.lvclass">, "error out"=w806:errorcluster)  [unwired: 14 in]
                    n375 = call-dynamic "externalSetParam.vi"("reference"=w807, "bentStyle"=BentStyleType."STRAIGHT", "error in (no error)"=w806, "setParam"=ExternaSetParamType."BendType") -> ("reference out"=w800:refnum<class "ClassRelationshipEdge.lvclass">, "error out"=w799:errorcluster)  [unwired: 14 in]
                    n376 = Build Array (concatenate)(w816, w800) -> (w815:refnum<class "AbstractEdge.lvclass">[])
                  }
                  frame -1 {
                  }
                }
              }
            }
            n377 = Bundle By Name(cluster=w763, "edges"=w764) -> (w765:T3)
            n378 = call <resource>:"CommonVIs_TimingLogger2.vi"("error in (no error)"=w754) -> ("error out"=w753:errorcluster)  [unwired: 10 in]
          }
          frame "CreateTypeDefEdgesFromTypeDefs" {
            n379 = Unbundle By Name(w831) -> ("edges"=w830:refnum<class "AbstractEdge.lvclass">[], "TypeDefs"=w826:T11[])
            n380 = Unbundle By Name(w831) -> ("nodes"=w828:refnum<class "ClassNode.lvclass">[], "classInfos"=w829:T4[], "TypeDefs"=w823:T11[])
            n381 = Array Size(array=w829) -> (size(s)=w827:i32)
            n382 = Array Subset(array=w828, index=w827) -> (w824:refnum<class "ClassNode.lvclass">[])  [unwired: 1 in]
            n383 = for {
              shift-right: [w838] -> w822
              shift-left: w834 -> [w837]
              tunnel: w824 -> [w836] mode=indexing
              tunnel: w823 -> [w842]
              tunnel: w824 -> [w835]
              shift-right: [w839] -> w832
              shift-left: w830 -> [w840]
              tunnel: w826 -> [w843] mode=indexing
              # "Association"
              n384 = Unbundle By Name(w843) -> ("TypeDefName"=w841:string)
              n385 = for {
                tunnel: w842 -> [w854] mode=indexing
                tunnel: w841 -> [w852]
                shift-right: [w850] -> w839
                shift-left: w840 -> [w851]
                shift-right: [w845] -> w838
                shift-left: w837 -> [w848]
                tunnel: [w848] -> _ mode=indexing
                tunnel: w836 -> [w847]
                tunnel: w835 -> [w846] mode=indexing
                n386 = Unbundle By Name(w854) -> ("TypeDefAttribInfo"=w844:T6[])
                n387 = for {
                  tunnel: [w879] -> w853 mode=indexing
                  tunnel: w844 -> [w878] mode=indexing
                  n388 = Unbundle By Name(w878) -> ("typeName"=w879:string)
                }
                n389 = Search 1D Array(1D array=w853, element=w852) -> (index of element=w849:i32)  [unwired: 1 out]
                n390 = case shown="0, Default" w849 {
                  tunnel: w847 -> [w875 _]
                  tunnel: [w857 w876] -> w845
                  tunnel: w846 -> [w855 _]
                  tunnel: w851 -> [w874 w877]
                  tunnel: [w873 w877] -> w850
                  tunnel: w848 -> [w856 w876]
                  frame 0, Default {
                    n391 = call <resource>:"ClassRelationshipEdge_Create.vi"("error in (no error)"=w856) -> ("reference out"=w872:refnum<class "ClassRelationshipEdge.lvclass">, "error out"=w871:errorcluster)  [unwired: 1 in, 16 out]
                    n392 = call-dynamic "externalSetParam.vi"("reference"=w872, "node"=w875, "error in (no error)"=w871, "setParam"=ExternaSetParamType."EndNode") -> ("reference out"=w869:refnum<class "ClassRelationshipEdge.lvclass">, "error out"=w868:errorcluster)  [unwired: 14 in]
                    n393 = call-dynamic "externalSetParam.vi"("reference"=w869, "node"=w855, "error in (no error)"=w868, "setParam"=ExternaSetParamType."StartNode") -> ("reference out"=w867:refnum<class "ClassRelationshipEdge.lvclass">, "error out"=w866:errorcluster)  [unwired: 14 in]
                    n394 = call-dynamic "externalSetParam.vi"("reference"=w867, "arrowHead"=ArrowHeadType."V", "error in (no error)"=w866, "setParam"=ExternaSetParamType."EndArrow") -> ("reference out"=w865:refnum<class "ClassRelationshipEdge.lvclass">, "error out"=w864:errorcluster)  [unwired: 14 in]
                    n395 = call-dynamic "externalSetParam.vi"("reference"=w865, "bentStyle"=BentStyleType."STRAIGHT", "error in (no error)"=w864, "setParam"=ExternaSetParamType."BendType") -> ("reference out"=w858:refnum<class "ClassRelationshipEdge.lvclass">, "error out"=w857:errorcluster)  [unwired: 14 in]
                    n396 = Build Array (concatenate)(w874, w858) -> (w873:refnum<class "AbstractEdge.lvclass">[])
                  }
                  frame -1 {
                  }
                }
              }
            }
            n397 = Bundle By Name(cluster=w831, "edges"=w832) -> (w833:T3)
            n398 = call <resource>:"CommonVIs_TimingLogger2.vi"("error in (no error)"=w822) -> ()  [unwired: 10 in, 1 out]
          }
          frame "GetBounds" {
            w898 = 10.0 ("gridX")
            n399 = call <resource>:"Graphics_Create.vi"("screenRef"="screenRef", "error in (no error)"=w901) -> ("reference out"=w891:refnum<class "Graphics.lvclass">, "error out"=w894:errorcluster)  [unwired: 1 in, 15 out]
            n400 = Unbundle By Name(w904) -> ("graph"=w896:refnum<class "Graph.lvclass">, "nodes"=w888:refnum<class "ClassNode.lvclass">[])
            n401 = Array Size(array=w888) -> (size(s)=w887:i32)
            n402 = call <resource>:"setFont.vi"("reference"=w891, "fontType"=LvFontType."User-specified Font", "font"=w893, "error in (no error)"=w894) -> ("reference out"=w889:refnum<class "Graphics.lvclass">, "error out"=w890:errorcluster)  [unwired: 14 out]
            n403 = Less Or Equal?(x=w887, y=7) -> (x <= y?=w885:bool)
            n404 = case shown="False" w885 {
              selector: w885 -> [_ w913]
              tunnel: [w906 w913] -> w884
              frame False {
                n405 = disable-structure shown="Disabled" {
                  disable-tunnel: [w907 FALSE] -> w906
                  frame Disabled {
                    n406 = Two Button Dialog(message="Since there are many classes to be shown\non the diagram, the methods and attribute has been hidden.\nTo show all classes attributes and methods, right click\non diagram and select \"Show all methods/attributes\"", 1:"Show anyway" ("F button name (\"Cancel\")"), 2:"Continue" ("T button name (\"OK\")")) -> (T button?=w908:bool)
                    n407 = Not(x=w908) -> (.not. x?=w907:bool)
                  }
                  frame Enabled {
                  }
                }
              }
              frame True {
              }
            }
            n408 = call <resource>:"Grid_Create.vi"("error in (no error)"=w890) -> ("reference out"=w899:refnum<class "Grid.lvclass">, "error out"=w902:errorcluster)  [unwired: 2 in, 15 out]
            n409 = call <resource>:"setGrid.vi"("reference"=w899, "gridX"=w898, "gridY"=w898, "error in (no error)"=w902) -> ("reference out"=w895:refnum<class "Grid.lvclass">, "error out"=w897:errorcluster)  [unwired: 14 out]
            n410 = for {
              shift-right: [w932] -> w883
              shift-left: w897 -> [w935]
              tunnel: w888 -> [w924] mode=indexing
              tunnel: [w936] -> w903 mode=indexing
              tunnel: w884 -> [w934]
              tunnel: w884 -> [w933]
              tunnel: w896 -> [w927]
              tunnel: w889 -> [w926]
              tunnel: w895 -> [w925]
              n411 = call <resource>:"ExternalGetParam.vi"("reference"=w924, "setParameter"=ExternalSetTypes."Methods") -> ("string"=w922:string)  [unwired: 12 in, 5 out]
              n412 = Spreadsheet String To Array(delimiter (Tab)="\n", format string="%s", spreadsheet string=w922, array type (2D Dbl)=string[] []) -> (array=w919:string[])
              n413 = Array Size(array=w919) -> (size(s)=w917:i32)
              n414 = Less Or Equal?(x=w917, y=12) -> (x <= y?=w914:bool)
              n415 = And(x=w933, y=w914) -> (x .and. y?=w915:bool)
              n416 = call <resource>:"SetVisibillitySettings.vi"("reference"=w924, "showAttribute"=w934, "showMethods"=w915, "error in (no error)"=w935) -> ("reference out"=w931:refnum<class "ClassNode.lvclass">, "error out"=w930:errorcluster)  [unwired: 14 out]
              n417 = call-dynamic "layout.vi"("reference"=w931, "graph"=w927, "graphics"=w926, "grid"=w925, "error in (no error)"=w930) -> ("reference out"=w929:refnum<class "ClassNode.lvclass">, "error out"=w928:errorcluster)  [unwired: 13 in]
              n418 = call-dynamic "getBounds.vi"("reference"=w929, "error in (no error)"=w928) -> ("bounds"=w936:T10, "error out"=w932:errorcluster)  [unwired: 15 in, 1 out]
            }
            n419 = Bundle By Name(cluster=w904, "bounds"=w903, "graphics"=w889, "grid"=w895) -> (w905:T3)
            n420 = call <resource>:"UMLEditor ControlBusyDialog.vi"("Title/StatusText"="Positioning classes", "error in (no error)"=w883) -> ("error out"=w880:errorcluster)  [unwired: 2 in, 15 out]
            n421 = call <resource>:"CommonVIs_TimingLogger2.vi"("error in (no error)"=w880) -> ()  [unwired: 10 in, 1 out]
          }
          frame "CheckInheritance" {
            n422 = Unbundle By Name(w947) -> ("nodesDone"=w937:i32[], "classInfos"=w952:T4[])
            n423 = for {
              tunnel: w952 -> [w979] mode=indexing
              tunnel: [w990] -> w948 mode=indexing
              tunnel: w937 -> [w988]
              tunnel: [w978] -> w941 mode=indexing
              i -> [w991]
              n424 = Unbundle By Name(w979) -> ("classPath"=w978:path)
              n425 = Unbundle By Name(w979) -> ("classPath"=w980:path)
              n426 = Unbundle By Name(w979) -> ("baseClasses"=w982:path[])
              n427 = Array Size(array=w982) -> (size(s)=w985:i32)
              n428 = Search 1D Array(1D array=w988, element=w991) -> (index of element=w987:i32)  [unwired: 1 out]
              n429 = Decrement(x=w985) -> (x-1=w989:i32)
              n430 = Index Array(array=w982, index=w989) -> ()  [unwired: 1 out]
              n431 = Greater Or Equal To 0?(x=w987) -> (x >= 0?=w986:bool)
              n432 = Build Array (concatenate)(w980, w982) -> (w981:path[])
              n433 = Select(t=-1, s=w986, f=w985) -> (s? t:f=w984:i32)
              n434 = Bundle("t"=w984, w991, w981) -> (w990:cluster{"t":i32, i32, path[]})  [unwired: 1 out]
            }
            n435 = Sort 1D Array(array=w948) -> (sorted array=w949:cluster{"t":i32, i32, path[]}[])
            n436 = Reverse 1D Array(array=w949) -> (reversed array=w946:cluster{"t":i32, i32, path[]}[])
            n437 = Index Array(array=w946) -> (element=w945:cluster{"t":i32, i32, path[]})  [unwired: 1 in]
            n438 = Unbundle(w945) -> ("t"=w944:i32, w940:path[])  [unwired: 1 out]
            n439 = for {
              tunnel: w941 -> [w962]
              tunnel: w940 -> [w961] mode=indexing
              shift-right: [w959] -> w938
              shift-left: i32[] [] -> [w960]
              tunnel: w937 -> [w958]
              n440 = Search 1D Array(1D array=w962, element=w961) -> (index of element=w957:i32)  [unwired: 1 out]
              n441 = Search 1D Array(1D array=w958, element=w957) -> (index of element=w954:i32)  [unwired: 1 out]
              n442 = Less Than 0?(x=w954) -> (x < 0?=w953:bool)
              n443 = Greater Or Equal To 0?(x=w957) -> (x >= 0?=w956:bool)
              n444 = And(x=w953, y=w956) -> (x .and. y?=w955:bool)
              n445 = case shown="False" w955 {
                tunnel: w960 -> [w965 w966]
                tunnel: [w964 w966] -> w959
                tunnel: w957 -> [w963 _]
                frame True {
                  n446 = Build Array (concatenate)(w965, w963) -> (w964:i32[])
                }
                frame False {
                }
              }
            }
            n447 = Greater Than 0?(x=w944) -> (x > 0?=w943:bool)
            n448 = case shown="True" w943 {
              tunnel: [w968 w977] -> w951
              tunnel: w947 -> [w968 w976]
              tunnel: ["CalcOtherPositions" ("y") w970] -> w942
              tunnel: w938 -> [_ w975]
              frame False {
              }
              frame True {
                n449 = Delete From Array(array=w975) -> (deleted portion=w973:i32)  [unwired: 2 in, 1 out]
                n450 = Less Than 0?(x=w973) -> (x < 0?=w972:bool)
                n451 = Build Array(w973) -> (w974:i32[])
                n452 = Bundle By Name(cluster=w976, "nodesToUse"=w974) -> (w977:T3)
                n453 = Select(t="CalcOtherPositions" ("y"), s=w972, f="CalcInheritancePos" ("y")) -> (s? t:f=w970:string)
              }
            }
          }
          frame "CalcInheritancePos" {
            w1002 = 0 ("startYpos")
            w1016 = 60  # heightGap
            w1011 = 20  # widthGap
            n454 = Unbundle By Name(w1019) -> ("nodesDone"=w1026:i32[], "nodesToUse"=w1021:i32[], "block"=w1006:cluster{"nodesInd":i32[], "bounds":T10}[])  [unwired: 1 out]
            n455 = Multiply(x=w1011, y=2) -> (x*y=w1009:i32)
            n456 = Index Array(array=w1021) -> (element=w1018:i32)  [unwired: 1 in]
            n457 = Array Size(array=w1006) -> (size(s)=w1008:i32)
            n458 = Reverse 1D Array(array=w1006) -> (reversed array=w1005:cluster{"nodesInd":i32[], "bounds":T10}[])
            n459 = call <resource>:"UMLEditor reversedEngineeringRecursiveInheritInfo.vi"("localIn"=w1019, "nodeIndex"=w1018, "widthGap"=w1011, "heightGap"=50, "error in (no error)"=w1020, "allInheritorIn"=i32[] []) -> ("BlockHeight"=w1001:i32, "width"=w1000:i32, "allInheritor"=w1017:i32[], "error out"=w994:errorcluster)  [unwired: 10 out]
            n460 = Index Array(array=w1006) -> (element=w1013:cluster{"nodesInd":i32[], "bounds":T10})  [unwired: 1 in]
            n461 = Index Array(array=w1005) -> (element=w1004:cluster{"nodesInd":i32[], "bounds":T10})  [unwired: 1 in]
            n462 = Unbundle By Name(w1004) -> ("bounds.x"=w999:dbl, "bounds.width"=w998:dbl)
            n463 = Multiply(x=w1008, y=w1009) -> (x*y=w1007:i32)
            n464 = call <resource>:"CommonVIs_TimingLogger2.vi"("error in (no error)"=w994) -> ("error out"=w993:errorcluster)  [unwired: 10 in]
            n465 = Add(x=w999, y=w998) -> (x+y=w997:dbl)
            n466 = Build Array (concatenate)(w1018, w1017) -> (w1012:i32[])
            n467 = Add(x=w997, y=w1007) -> (x+y=w1003:dbl)
            n468 = call <resource>:"UMLEditor reversedEngineeringRecursiveSetPos.vi"("BlockXpos"=w1003, "startYpos"=w1002, "nodeIndex"=w1018, "widthGap"=w1011, "heightGap"=w1016, "error in (no error)"=w993, "localIn"=w1019) -> ("localOut"=w1015:T3, "error out"=w992:errorcluster)  [unwired: 11 out]
            n469 = call <resource>:"CommonVIs_TimingLogger2.vi"("error in (no error)"=w992) -> ()  [unwired: 10 in, 1 out]
            n470 = Bundle By Name(cluster=w1013, "nodesInd"=w1012, "bounds.x"=w1003, "bounds.y"=w1002, "bounds.width"=w1000, "bounds.height"=w1001) -> (w1014:cluster{"nodesInd":i32[], "bounds":T10})
            n471 = Build Array (concatenate)(w1026, w1012) -> (w1024:i32[])
            n472 = Build Array (concatenate)(w1006, w1014) -> (w1023:cluster{"nodesInd":i32[], "bounds":T10}[])
            n473 = Bundle By Name(cluster=w1015, "nodesDone"=w1024, "block"=w1023) -> (w1025:T3)
          }
          frame "CalcOtherPositions" {
            w1033 = 80  # heightGap
            w1038 = 20  # widthGap
            n474 = Unbundle By Name(w1037) -> ("nodesDone"=w1036:i32[], "bounds"=w1035:T10[], "block"=w1041:cluster{"nodesInd":i32[], "bounds":T10}[])
            n475 = Multiply(x=w1038, y=3) -> (x*y=w1043:i32)
            n476 = Reverse 1D Array(array=w1041) -> (reversed array=w1040:cluster{"nodesInd":i32[], "bounds":T10}[])
            n477 = Array Size(array=w1041) -> (size(s)=w1042:i32)
            n478 = Index Array(array=w1040) -> (element=w1039:cluster{"nodesInd":i32[], "bounds":T10})  [unwired: 1 in]
            n479 = Unbundle By Name(w1039) -> ("bounds.x"=w1029:dbl, "bounds.width"=w1030:dbl)
            n480 = Multiply(x=w1042, y=w1043) -> (x*y=w1031:i32)
            n481 = Compound Arithmetic op=ADD(w1029, w1030, w1031) -> (w1028:dbl)
            n482 = for {
              tunnel: w1036 -> [w1055]
              tunnel: w1035 -> [w1052] mode=indexing
              tunnel: [w1051] -> w1034 mode=indexing
              shift-right: [w1047] -> _
              shift-left: 0.0 -> [w1049]
              tunnel: w1028 -> [w1050]
              tunnel: w1033 -> [w1048]
              i -> [w1054]
              n483 = Search 1D Array(1D array=w1055, element=w1054) -> (index of element=w1053:i32)  [unwired: 1 out]
              n484 = case shown="-1" w1053 {
                tunnel: w1052 -> [w1061 w1065]
                tunnel: [w1063 w1065] -> w1051
                tunnel: w1050 -> [w1062 _]
                tunnel: w1049 -> [w1060 w1064]
                tunnel: w1048 -> [w1057 _]
                tunnel: [w1056 w1064] -> w1047
                frame -1 {
                  n485 = Unbundle By Name(w1061) -> ("height"=w1059:dbl)
                  n486 = Add(x=w1060, y=w1059) -> (x+y=w1058:dbl)
                  n487 = Add(x=w1058, y=w1057) -> (x+y=w1056:dbl)
                  n488 = Bundle By Name(cluster=w1061, "x"=w1062, "y"=w1060) -> (w1063:T10)
                }
                frame 0.., Default {
                }
              }
            }
            n489 = Bundle By Name(cluster=w1037, "bounds"=w1034) -> (w1046:T3)
          }
          frame "SetPos" {
            n490 = Unbundle By Name(w1075) -> ("edges"=w1068:refnum<class "AbstractEdge.lvclass">[], "graph"=w1071:refnum<class "Graph.lvclass">, "nodes"=w1074:refnum<class "ClassNode.lvclass">[], "bounds"=w1072:T10[], "graphics"=w1070:refnum<class "Graphics.lvclass">, "grid"=w1069:refnum<class "Grid.lvclass">)
            n491 = for {
              tunnel: w1074 -> [w1094] mode=indexing
              shift-right: [w1088] -> w1067
              shift-left: w1073 -> [w1093]
              tunnel: w1072 -> [w1092] mode=indexing
              tunnel: w1071 -> [w1086]
              tunnel: w1070 -> [w1085]
              tunnel: w1069 -> [w1084]
              n492 = Unbundle By Name(w1092) -> ("x"=w1091:dbl, "y"=w1090:dbl)
              n493 = call <resource>:"setPosition.vi"("reference"=w1094, "x"=w1091, "y"=w1090, "error in (no error)"=w1093) -> ("reference out"=w1089:refnum<class "ClassNode.lvclass">, "error out"=w1087:errorcluster)  [unwired: 1 in, 13 out]
              n494 = call-dynamic "layout.vi"("reference"=w1089, "graph"=w1086, "graphics"=w1085, "grid"=w1084, "error in (no error)"=w1087) -> ("error out"=w1088:errorcluster)  [unwired: 13 in, 1 out]
            }
            n495 = for {
              tunnel: w1068 -> [w1082] mode=indexing
              shift-right: [w1077] -> w1066
              shift-left: w1067 -> [w1078]
              n496 = To More Specific Class(target class=refnum<class "SegmentedLineEdge.lvclass"> refnum ("reference"), reference=w1082, error in=w1078) -> (specific class reference=w1080:refnum<class "SegmentedLineEdge.lvclass">, error out=w1079:errorcluster)
              n497 = call <resource>:"SetSplitWireIfLongDistance.vi"("reference"=w1080, "MaxLength"=1500.0, "error in (no error)"=w1079) -> ("error out"=w1077:errorcluster)  [unwired: 16 out]
            }
            n498 = call <resource>:"CommonVIs_TimingLogger2.vi"("error in (no error)"=w1066) -> ()  [unwired: 10 in, 1 out]
          }
          frame "TranslateAplicationNodes?" {
            n499 = Unbundle By Name(w1111) -> ("graph"=w1097:refnum<class "Graph.lvclass">, "nodes"=w1109:refnum<class "ClassNode.lvclass">[], "graphics"=w1099:refnum<class "Graphics.lvclass">, "grid"=w1098:refnum<class "Grid.lvclass">)  [unwired: 1 out]
            n500 = local read "ApplicationNodes"() -> (w1103:i32[])
            n501 = for {
              tunnel: w1103 -> [w1133] mode=indexing
              tunnel: w1109 -> [w1134]
              shift-right: [w1126] -> _
              shift-left: 0.0 -> [w1125]
              tunnel: [w1130] -> w1107 mode=indexing
              tunnel: [w1124] -> w1096 mode=indexing
              tunnel: [w1123] -> w1102 mode=indexing
              n502 = Index Array(array=w1134, index=w1133) -> (element=w1123:refnum<class "ClassNode.lvclass">)
              n503 = call-dynamic "getBounds.vi"("reference"=w1123) -> ("bounds"=w1132:T10)  [unwired: 16 in, 2 out]
              n504 = Add(x=50.0, y=w1125) -> (x+y=w1127:dbl)
              n505 = call <resource>:"Rectangel GetRectInfo.vi"("bounds"=w1132) -> ("maxX"=w1129:dbl, "maxY"=w1130:dbl)  [unwired: 1 in, 16 out]
              n506 = Bundle By Name(cluster=w1132, "x"=w1125, "y"=0.0) -> (w1124:T10)
              n507 = Add(x=w1127, y=w1129) -> (x+y=w1126:dbl)
            }
            n508 = Array Max & Min(array=w1107) -> (max value=w1106:dbl)  [unwired: 3 out]
            n509 = Add(x=50.0, y=w1106) -> (x+y=w1104:dbl)
            n510 = for {
              shift-right: [w1121] -> w1100
              shift-left: w1101 -> [w1122]
              tunnel: w1097 -> [w1120]
              tunnel: w1099 -> [w1119]
              tunnel: w1098 -> [w1118]
              tunnel: w1102 -> [w1117] mode=indexing
              tunnel: w1096 -> [w1116] mode=indexing
              n511 = Unbundle(w1116) -> ("x"=w1113:dbl, "y"=w1112:dbl)  [unwired: 2 out]
              n512 = call <resource>:"setPosition.vi"("reference"=w1117, "x"=w1113, "y"=w1112, "error in (no error)"=w1122) -> ("reference out"=w1114:refnum<class "ClassNode.lvclass">, "error out"=w1115:errorcluster)  [unwired: 1 in, 13 out]
              n513 = call-dynamic "layout.vi"("reference"=w1114, "graph"=w1120, "graphics"=w1119, "grid"=w1118, "error in (no error)"=w1115) -> ("error out"=w1121:errorcluster)  [unwired: 13 in, 1 out]
            }
            n514 = for {
              tunnel: w1109 -> [w1144] mode=indexing
              shift-right: [w1142] -> w1095
              shift-left: w1100 -> [w1143]
              tunnel: w1097 -> [w1141]
              tunnel: w1099 -> [w1140]
              tunnel: w1098 -> [w1139]
              tunnel: w1104 -> [w1138]
              tunnel: w1103 -> [w1137]
              i -> [w1136]
              n515 = Search 1D Array(1D array=w1137, element=w1136) -> (index of element=w1135:i32)  [unwired: 1 out]
              n516 = case shown="-1" w1135 {
                tunnel: w1144 -> [_ w1155]
                tunnel: w1143 -> [w1145 w1154]
                tunnel: [w1145 w1152] -> w1142
                tunnel: w1141 -> [_ w1150]
                tunnel: w1140 -> [_ w1149]
                tunnel: w1139 -> [_ w1148]
                tunnel: w1138 -> [_ w1147]
                frame 0, Default {
                }
                frame -1 {
                  n517 = call-dynamic "translate.vi"("reference"=w1155, "dx"=0.0, "dy"=w1147, "error in (no error)"=w1154) -> ("reference out"=w1153:refnum<class "ClassNode.lvclass">, "error out"=w1151:errorcluster)  [unwired: 14 in]
                  n518 = call-dynamic "layout.vi"("reference"=w1153, "graph"=w1150, "graphics"=w1149, "grid"=w1148, "error in (no error)"=w1151) -> ("error out"=w1152:errorcluster)  [unwired: 13 in, 1 out]
                }
              }
            }
            n519 = call <resource>:"CommonVIs_TimingLogger2.vi"("error in (no error)"=w1095) -> ()  [unwired: 10 in, 1 out]
          }
          frame "CreateDiagram" {
            n520 = Unbundle By Name(w1168) -> ("edges"=w1167:refnum<class "AbstractEdge.lvclass">[], "nodes"=w1161:refnum<class "ClassNode.lvclass">[])
            n521 = call <resource>:"ClassDiagramGraph_Create.vi"("error in (no error)"=w1170) -> ("reference out"=w1172:refnum<class "ClassDiagramGraph.lvclass">, "error out"=w1171:errorcluster)  [unwired: 1 in, 16 out]
            n522 = call-dynamic "setNodes.vi"("reference"=w1172, "nodes"=w1161, "error in (no error)"=w1171) -> ("reference out"=w1175:refnum<class "ClassDiagramGraph.lvclass">, "error out"=w1174:errorcluster)  [unwired: 15 in]
            n523 = call-dynamic "setEdges.vi"("reference"=w1175, "edges"=w1167, "error in (no error)"=w1174) -> ("reference out"=w1173:refnum<class "ClassDiagramGraph.lvclass">, "error out"=w1158:errorcluster)  [unwired: 15 in]
            n524 = call <resource>:"CommonVIs_TimingLogger2.vi"("error in (no error)"=w1158) -> ("error out"=w1157:errorcluster)  [unwired: 10 in]
            n525 = call-dynamic "layout.vi"("reference"=w1173, "error in (no error)"=w1157) -> ("reference out"=w1169:refnum<class "ClassDiagramGraph.lvclass">, "error out"=w1160:errorcluster)  [unwired: 16 in]
            n526 = Bundle By Name(cluster=w1168, "graph"=w1169) -> (w1162:T3)
            n527 = Unbundle By Name(w1162) -> ("graphics"=w1165:refnum<class "Graphics.lvclass">, "grid"=w1164:refnum<class "Grid.lvclass">)
            n528 = call-dynamic "Destroy.vi"("reference"=w1164, "error in (no error)"=w1160) -> ("error out"=w1163:errorcluster)  [unwired: 16 in, 1 out]
            n529 = call-dynamic "Destroy.vi"("reference"=w1165, "error in (no error)"=w1163) -> ("error out"=w1156:errorcluster)  [unwired: 16 in, 1 out]
            n530 = case shown="False" w1159 {
              tunnel: ["XMI-CleanUp" ("y") "Exit" ("y")] -> w1166
              frame True {
              }
              frame False {
              }
            }
            n531 = call <resource>:"CommonVIs_TimingLogger2.vi"("error in (no error)"=w1156) -> ()  [unwired: 10 in, 1 out]
          }
          frame "XMI-CleanUp" {
            n532 = Unbundle By Name(w1184) -> ("nodes"=w1181:refnum<class "ClassNode.lvclass">[])
            n533 = call <vilib>:"Dflt Data Dir.vi"() -> ("App:Default Data Directory"=w1179:path)
            n534 = Build Path(base path=w1179, name or relative path="XMI_Import") -> (appended path=w1178:path)
            n535 = for {
              shift-right: [w1187] -> w1182
              shift-left: w1183 -> [w1188]
              tunnel: w1181 -> [w1186] mode=indexing
              tunnel: w1178 -> [_]
              n536 = call-dynamic "ExternalSetParam.vi"("reference"=w1186, "setParameter"=ExternalSetTypes."ClassPath", "error in (no error)"=w1188, "ClassPath"=path "") -> ("error out"=w1187:errorcluster)  [unwired: 14 in, 1 out]
            }
          }
        }
        n537 = Unbundle By Name(w57) -> ("status"=w56:bool)
        n538 = Equal?(x=w55, y="Exit") -> (x = y?=w53:bool)
        n539 = Or(x=w53, y=w56) -> (x .or. y?=w52:bool)
      }
    }
    frame Error {
    }
  }
  n540 = Unbundle By Name(w28) -> ("graph"=→"newCLassDiagram":refnum<class "Graph.lvclass">, "cancel"=w26:bool, "nodes"=w15:refnum<class "ClassNode.lvclass">[], "edges"=w27:refnum<class "AbstractEdge.lvclass">[])
  n541 = call <resource>:"ContextHelp_LeavingDialog.vi"("error in (no error)"=w2) -> ("error out"=w11:errorcluster)  [unwired: 18 out]
  n542 = property class="VI"(error in=w2, "Front Panel.Open"=FALSE ("Front Panel Window:Open")) -> (error out=→"error out":errorcluster)  [unwired: 1 in, 1 out]
  n543 = call <resource>:"CommonVIs_TimingLogger2.vi"("error in (no error)"=w2, "Name"="<<LOG>>") -> ()  [unwired: 9 in, 1 out]
  n544 = Empty Array?(array=w15) -> (empty?=w13:bool)
  n545 = call <resource>:"UMLEditor ControlBusyDialog.vi"("error in (no error)"=w11, "Action(SendStatusMessage)"=UMLEditor_BusyDialogAction."Close" ("Action")) -> ()  [unwired: 2 in, 16 out]
  n546 = Or(x=w26, y=w13) -> (x .or. y?=w14:bool)
  n547 = case shown="No Error" w2 {
    tunnel: w15 -> [_ w1195]
    tunnel: w27 -> [_ w1194]
    tunnel: w14 -> [w1192 _]
    tunnel: [w1192 TRUE ("canel")] -> w25
    frame No Error {
    }
    frame Error {
      n548 = for {
        tunnel: w1195 -> [w1197] mode=indexing
        n549 = call-dynamic "Destroy.vi"("reference"=w1197) -> ()  [unwired: 17 in, 2 out]
      }
      n550 = for {
        tunnel: w1194 -> [w1196] mode=indexing
        n551 = call-dynamic "Destroy.vi"("reference"=w1196) -> ()  [unwired: 18 in, 1 out]
      }
    }
  }
  "cancel" <- w25
